vi "SpectrometerSpinCoater_v07.vi"() -> ()   [LabVIEW 2018]
uses:
  <instrlib>/Classes/CCD/Abstract_CCD/Abstract_CCD.lvclass
  <instrlib>/Classes/SpinCoater/SpinCoater.lvclass
  TypDef/DeviceQueue_TypeDef.ctl
  TypDef/DeviceQueue_Action.ctl
  TypDef/DataQueue_TypeDef.ctl
  TypDef/DataQueue_Action.ctl
  <vilib>/Utility/error.llb/DialogType.ctl
  <instrlib>/Classes/CCD/Avantes/Avantes.lvclass
  C:/Program Files/National Instruments/LabVIEW 2018/instr.lib/Classes/CCD/Abstract_CCD/Abstract_CCD.lvclass
  <vilib>/Analysis/baseanly.llb/A x Vector.vi
  <vilib>/Analysis/NI_AALBase.lvlib
panel:
  out "Time.spin":refnum<file>
  out "Meas.spin":refnum<file>
  out "Arduino":bool
  out "NKT":bool
  out "Spectromter":bool
  in  "Abort Button":bool
  in  "Stop Button":bool
  in  "Tab Control":enum32{"Measure", "Settings"}(tab)
  in  "Program Spin Coater":T1(array[cluster])
  in  "Spectra Count":u16
  in  "Measure Spectrum":bool
  out "Action":string
  out "Overall Time":dbl
  in  "Seconds after Spin Stop":dbl[unit]=0.5
  in  "Seconds to Spin Start":dbl[unit]=1.0
  in  "Calculate Frames":bool=TRUE
  in  "Frames":i32
  in  "StartMeasurement_Button":bool
  in  "Preview":bool
  out "XY Graph":T2(graph)
  in  "Frames for Spectrometer":dbl=1.0
  in  "StartSpin_Button":bool
  in  "Record RefSpec":bool
  in  "Record_Darkspec":bool
  in  "Comments":string="Just for testing"
  in  "File Name":string="Temp"
  in  "Save Path":path=path "C:/Users/Timo/Desktop/SpinCoater/Measurement"
  out "Frame Rate":dbl[unit]
  in  "Integration Time":dbl[unit]=3e-05
  in  "Dividider Get Spectra":u32=1 min=1
  in  "Automatically \nadjust count":bool=TRUE
  in  "Reset Count\nafter Spin Coating":bool=TRUE
  in  "Speed":dbl
  in  "Milliseconds":dbl
  in  "Debug":bool
  in  "Port Arduino":refnum<visa-resource-name>="COM6"
  out "Error Arduino":bool caption="Error"
  in  "Init_Arduino":bool=TRUE caption="Init"
  out "Caption_Settings_Arduino":string="Arduino"
  out "Caption_Settings_NKT":string="NKT Laser"
  out "Error_Spectromter":bool caption="Error"
  in  "Init_Spectrometer":bool=TRUE caption="Init"
  out "Caption_Settings_Spectrometer":string="Spectromter"
  # "Speed (rpm)   Time (s)        Acceleration \n                                               (rpm/s)"
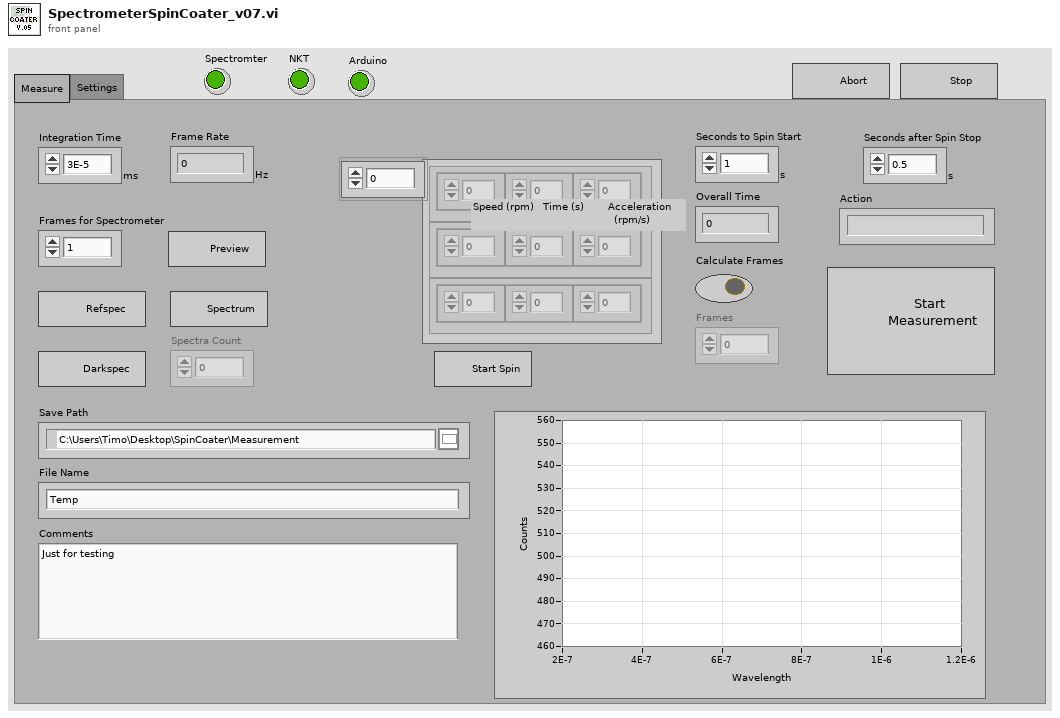
[diagram p1: front panel]
types:
  T1 = cluster{"Speed (rpm)":dbl, "Time (s)":dbl, "Acc (rpm/s)":dbl}[]
  T2 = cluster{"Wavlength":dbl[unit][], "Image":dbl[]}[]
  T3 = cluster{"Dark":cluster{"Image":dbl[][][], "Frame Size":cluster{"F":i32, "Y":i32, "X":i32}}[], "Ref":cluster{"Image":dbl[][][], "Frame Size":cluster{"F":i32, "Y":i32, "X":i32}}[], "Wavlength":dbl[unit][], "spec":dbl[][]}
  T4 = cluster{"Abstract_CCD.lvclass":refnum<class "Abstract_CCD.lvclass">, "SpinCoater.lvclass":refnum<class "SpinCoater.lvclass">}
  T5 = typedef "DataQueue_TypeDef.ctl" = cluster{"QueueAction":T6, "Data":cluster{"Image":dbl[][][], "Frame Size":cluster{"F":i32, "Y":i32, "X":i32}}[], "Data_Raw":cluster{"Image":dbl[][][], "Frame Size":cluster{"F":i32, "Y":i32, "X":i32}}[], "Data_Dark":cluster{"Image":dbl[][][], "Frame Size":cluster{"F":i32, "Y":i32, "X":i32}}[], "Data_Ref":cluster{"Image":dbl[][][], "Frame Size":cluster{"F":i32, "Y":i32, "X":i32}}[], "Device Information":string[], "Numeric Control":dbl, "Boolean":bool, "Wavelength":dbl[unit][], "Time":dbl[], "Time Stamp":timestamp, "Numeric Control 2":dbl}
  T6 = typedef "DataQueue_Action.ctl" = enum16{"TimeOut", "Close_Program", "Stop_Measurement", "Measure_InSituSpinCoating", "Measure_Spectrum", "Save_Data", "Set_Ref", "Set_Dark", "Set_Wavelength", "Spectrometer_Measure", "Spectrometer_Preview", "Transfer_Settings"}
  T7 = typedef "DeviceQueue_TypeDef.ctl" = cluster{"QueueAction":T8, "Numeric 1":dbl, "Numeric 2":dbl, "Boolean 1":bool, "Boolean 2":bool, "Spin Program":dbl[][], "Spin Prg v07":cluster{"Speed (rpm)":dbl, "Time (s)":dbl, "Acc (rpm/s)":dbl}[]}
  T8 = typedef "DeviceQueue_Action.ctl" = enum16{"TimeOut", "Close_Program", "Abort", "Spectrometer_Init", "Spectrometer_Close", "Spectrometer_DeviceInformation", "Spectrometer_Measure", "Spectrometer_Preview", "Spectrometer_Abort", "Spectrometer_StartMeasurement", "Spectrometer_GetData", "Spectrometer_StopMeasurement", "Spectrometer_SetIntegrationTime", "Spectrometer_SetFrames", "Spectrometer_SetDarkspec", "Spectrometer_SetReference", "Spectrometer_SetTriggerMode", "Laser_Init", "Laser_Close", "Arduino_Init", "Arduino_Close", "Arduino_LoadProgram", "Arduino_StartProgram", "Arduino_SetSpeed", "Arduino_SetMillis", "Arduino_StopSpin", "Measure_InSitu", "Measure_Spectrum", "Measure_Stop"}
  T9 = enum16{"open", "replace", "create", "open or create", "replace or create", "replace or create with confirmation"}
  T10 = cluster{"Image":dbl[][][], "Frame Size":cluster{"F":i32, "Y":i32, "X":i32}}[]
  T11 = cluster{"Image":dbl[][][], "Frame Size":cluster{"F":i32, "Y":i32, "X":i32}}
  T12 = cluster{"Wavlength":dbl[unit][], "A x Vector":dbl[]}
  T13 = cluster{"Wavlength":dbl[unit][], "A x Vector":dbl[]}[]
  T14 = cluster{u16[][], u16[][], dbl[], "Numeric Control":dbl, "Numeric Control 2":dbl}
  T15 = typedef "DialogType.ctl" = u16
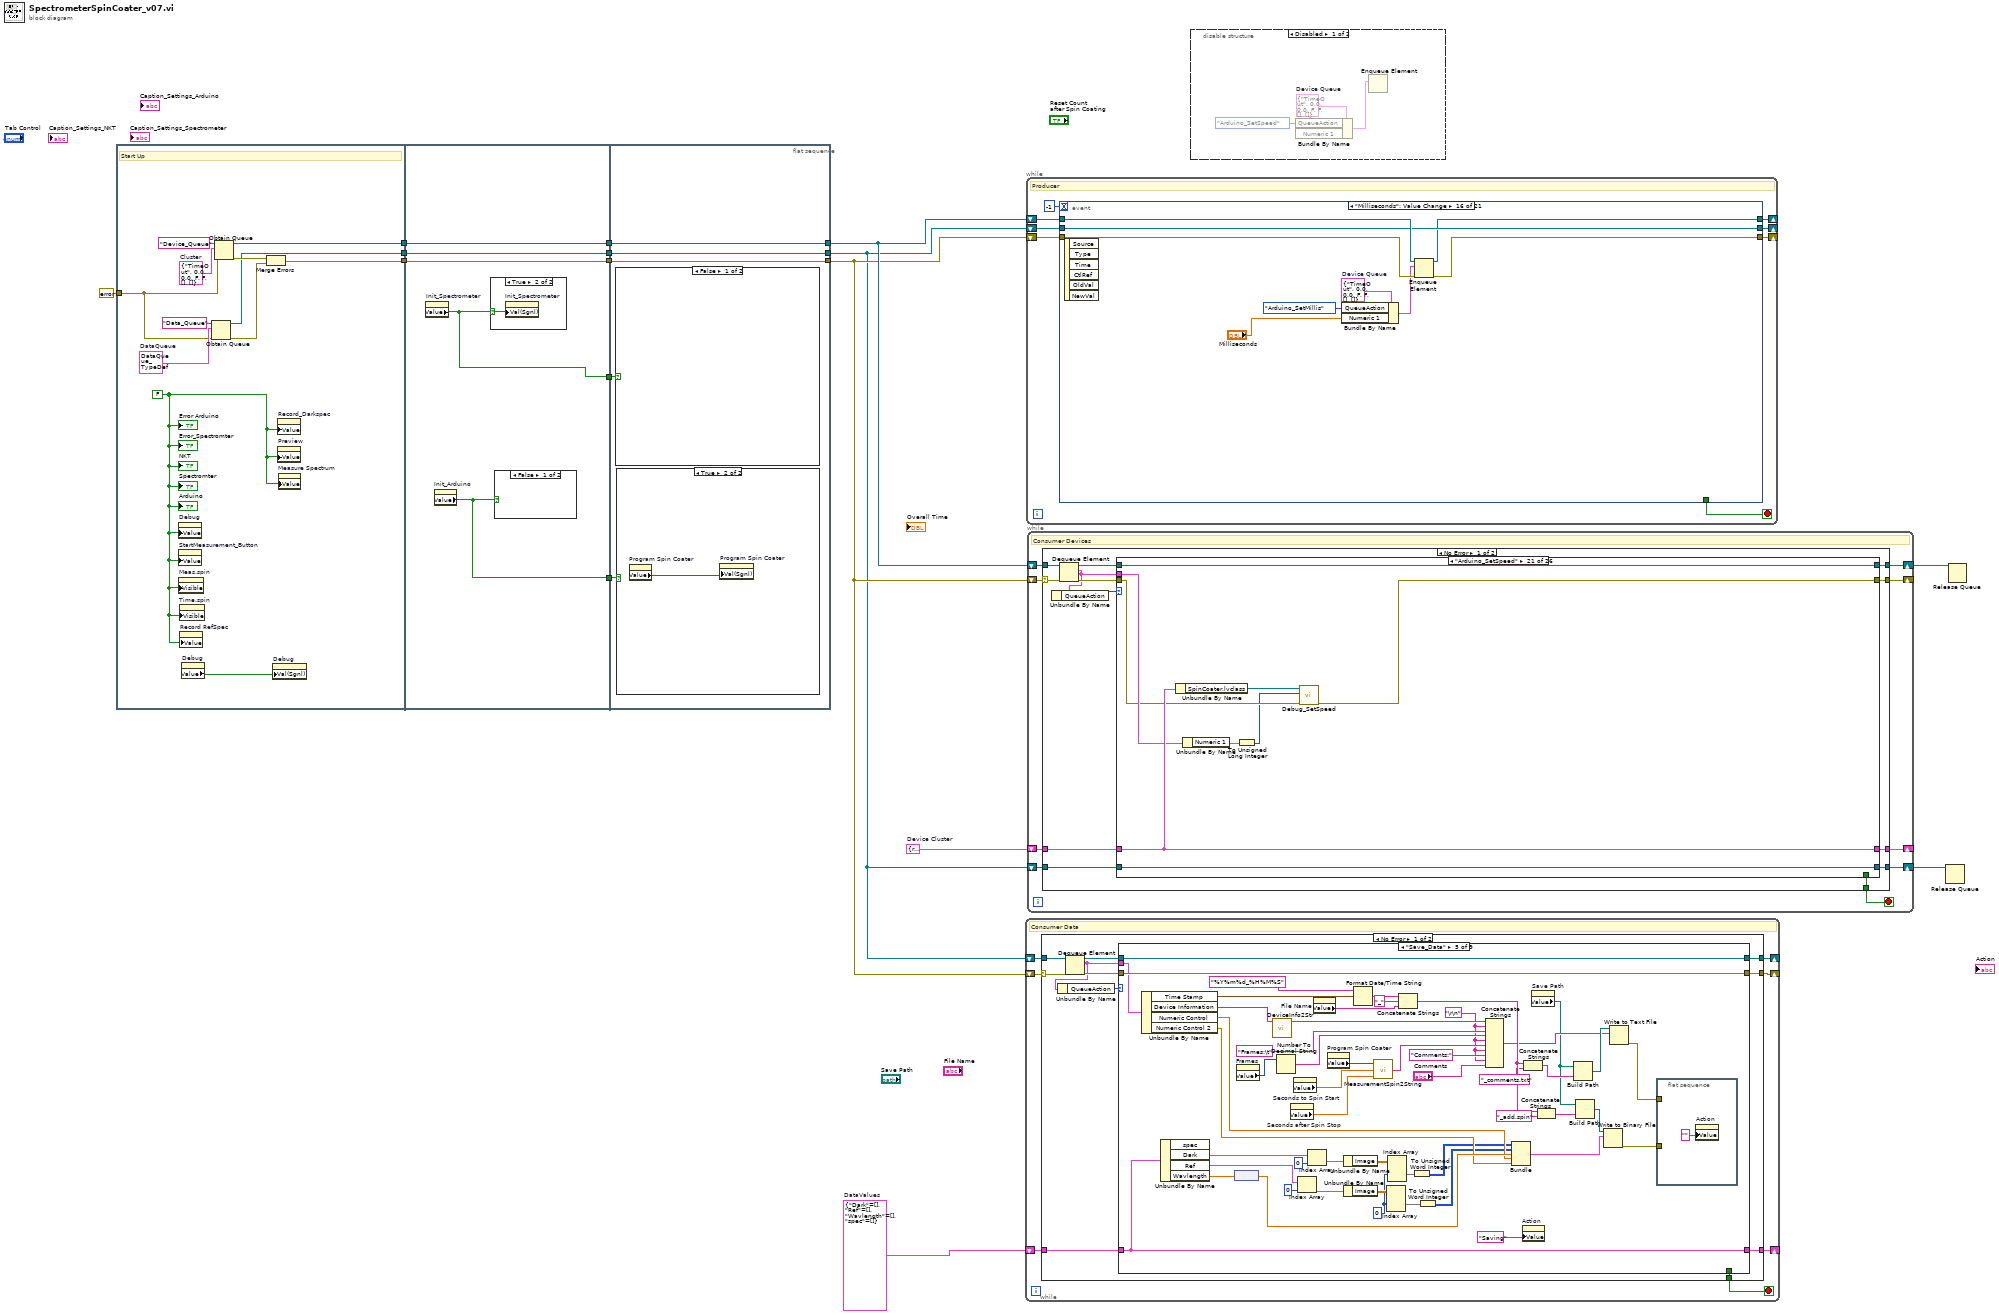
[diagram p0: block diagram]
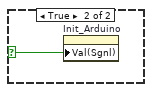
[diagram p3: hidden frame]
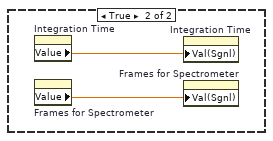
[diagram p6: hidden frame]
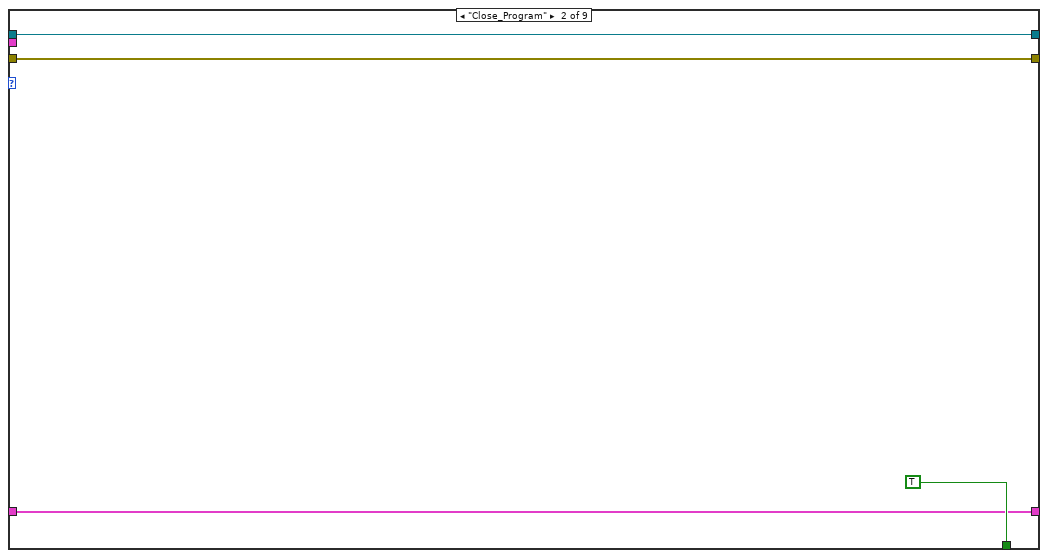
[diagram p8: hidden frame]
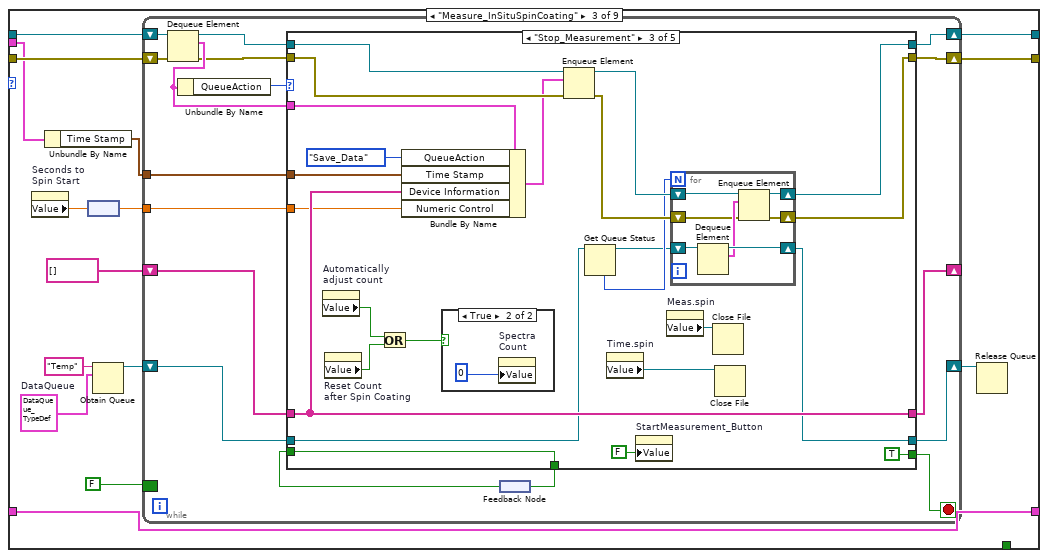
[diagram p9: hidden frame]
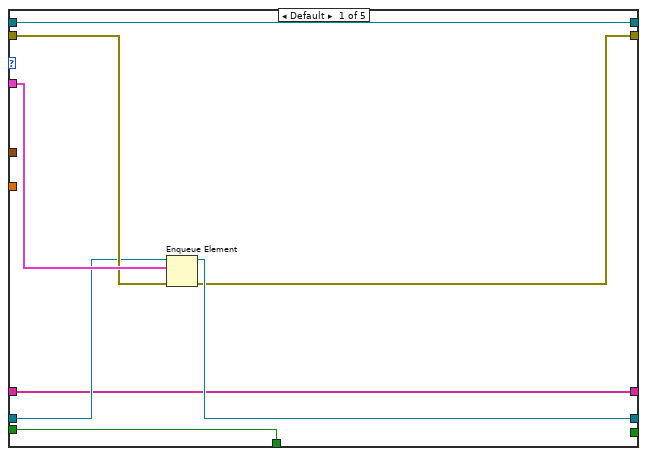
[diagram p10: hidden frame]
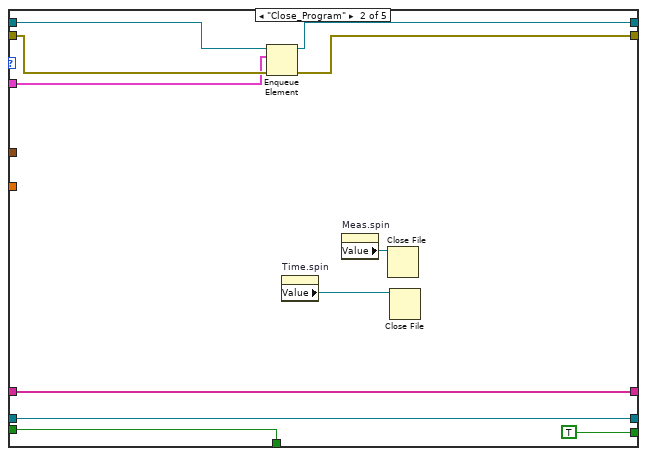
[diagram p11: hidden frame]
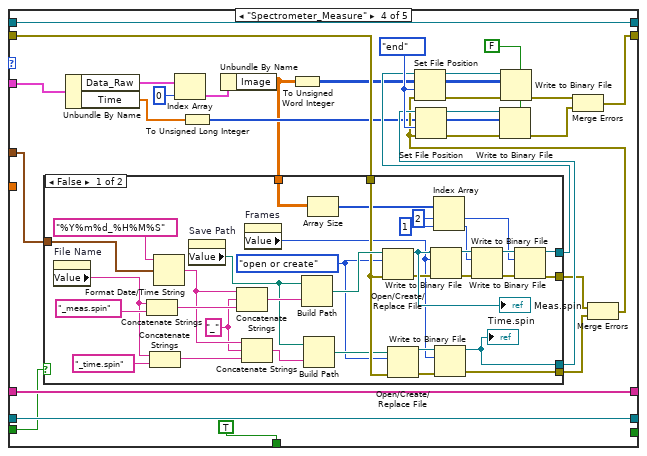
[diagram p13: hidden frame]
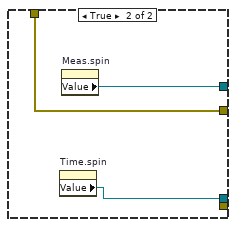
[diagram p14: hidden frame]
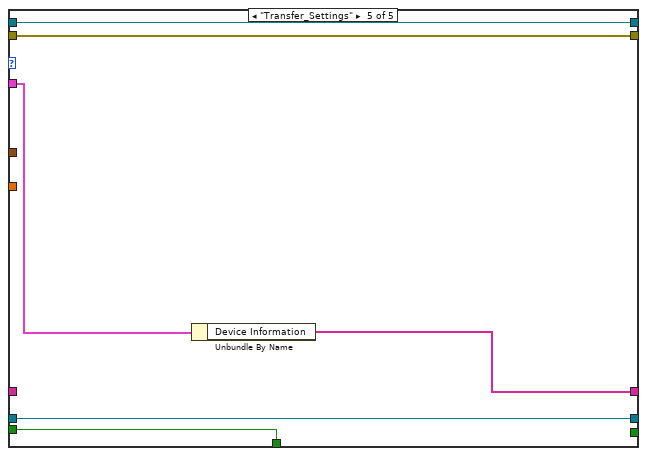
[diagram p15: hidden frame]
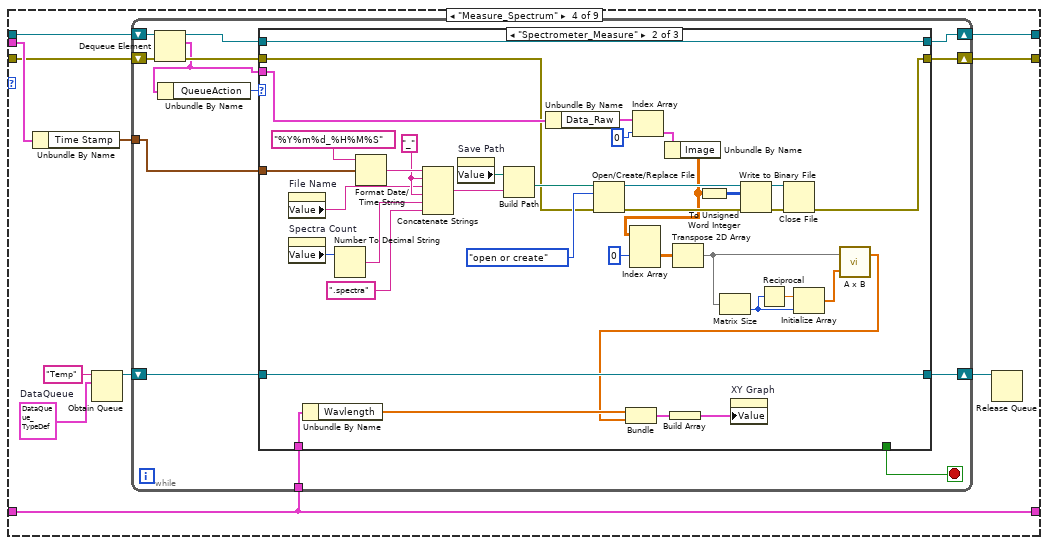
[diagram p16: hidden frame]
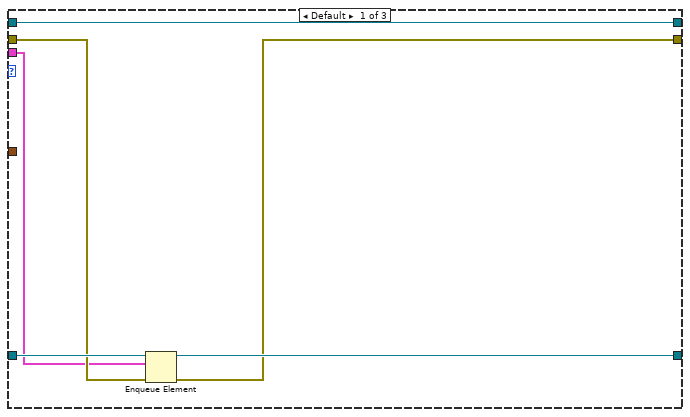
[diagram p17: hidden frame]
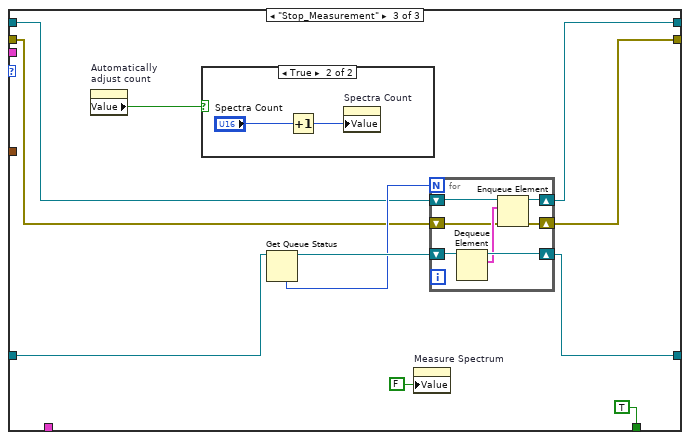
[diagram p18: hidden frame]
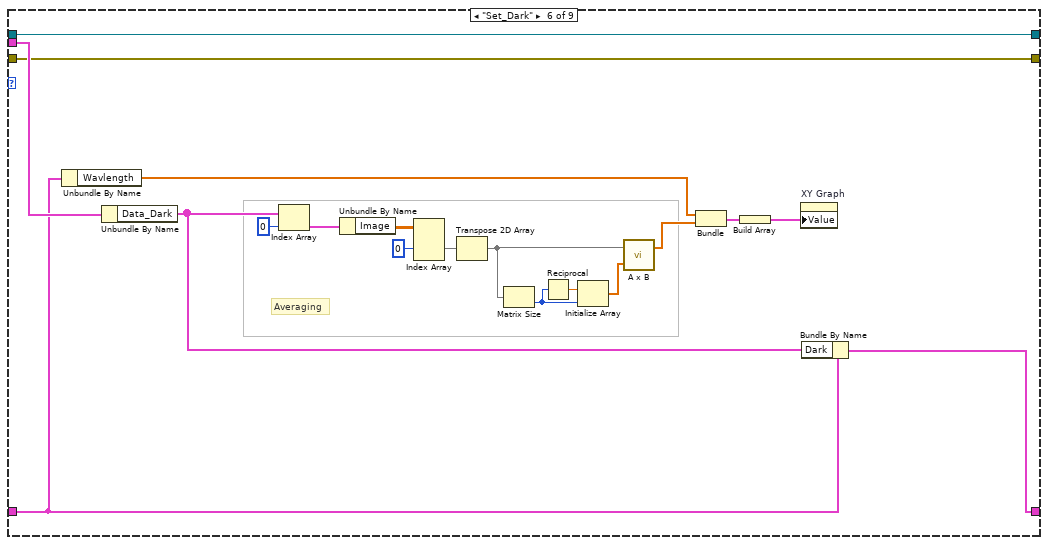
[diagram p20: hidden frame]
diagram:
  w6 = T3 {"Dark"=[], "Ref"=[], "Wavlength"=[], "spec"=[]}  # DataValues
  w11 = T4 {"Abstract_CCD.lvclass"=refnum, "SpinCoater.lvclass"=refnum}  # Device Cluster
  n1 = flat-sequence {
    tunnel: errorcluster {"status"=FALSE, "code"=0, "source"=""} ("error constant") -> [w23]
    tunnel: [w26] -> w15
    tunnel: [w20] -> w14
    tunnel: [w19] -> w13
    tunnel: w15 -> [w33]
    tunnel: w14 -> [w32]
    tunnel: w13 -> [w31]
    tunnel: [w33] -> w5
    tunnel: [w32] -> w4
    tunnel: [w31] -> w3
    tunnel: [w30] -> w2
    tunnel: [w29] -> w1
    tunnel: [w38] -> w8
    tunnel: [w39] -> w7
    tunnel: [w40] -> w12
    tunnel: w5 -> [w40]
    tunnel: w4 -> [w39]
    tunnel: w3 -> [w38]
    tunnel: w2 -> [w37]
    tunnel: w1 -> [w36]
    frame #0 {
      w24 = T5 {"QueueAction"=enum."TimeOut", "Data"=[], "Data_Raw"=[], "Data_Dark"=[], "Data_Ref"=[], "Device Information"=[], "Numeric Control"=0.0, "Boolean"=FALSE, "Wavelength"=[], "Time"=[], "Time Stamp"=timestamp(0 s since 1904-01-01), "Numeric Control 2"=0.0}  # DataQueue
      w27 = T7 {"QueueAction"=enum."TimeOut", "Numeric 1"=0.0, "Numeric 2"=0.0, "Boolean 1"=FALSE, "Boolean 2"=FALSE, "Spin Program"=[], "Spin Prg v07"=[]}  # Cluster
      w18 = FALSE ("Error Arduino")
      # "Start Up"
      n2 = property on="Debug" class="Bool (strict)"("Value"=w18) -> ()  [unwired: 2 in, 2 out]
      n3 = property on="StartMeasurement_Button" class="Bool (strict)"("Value"=w18) -> ()  [unwired: 2 in, 2 out]
      n4 = property on="Meas.spin" class="Ref (strict)"("Visible"=w18) -> ()  [unwired: 2 in, 2 out]
      n5 = property on="Time.spin" class="Ref (strict)"("Visible"=w18) -> ()  [unwired: 2 in, 2 out]
      n6 = property on="Record RefSpec" class="Bool (strict)"("Value"=w18) -> ()  [unwired: 2 in, 2 out]
      n7 = property on="Debug" class="Bool (strict)"() -> ("Value"=w17:bool)  [unwired: 2 in, 2 out]
      n8 = Obtain Queue(name (unnamed)="Data_Queue", element data type=w24, error in (no error)=w23) -> (queue out=w20:refnum<queue>, error out=w21:errorcluster)  [unwired: 2 in, 1 out]
      n9 = Obtain Queue(name (unnamed)="Device_Queue", element data type=w27, error in (no error)=w23) -> (queue out=w26:refnum<queue>, error out=w22:errorcluster)  [unwired: 2 in, 1 out]
      n10 = Merge Errors(w22, w21) -> (w19:errorcluster)
      n11 = property on="Debug" class="Bool (strict)"("Val(Sgnl)"=w17) -> ()  [unwired: 2 in, 2 out]
      n12 = property on="Record_Darkspec" class="Bool (strict)"("Value"=w18) -> ()  [unwired: 2 in, 2 out]
      n13 = property on="Preview" class="Bool (strict)"("Value"=w18) -> ()  [unwired: 2 in, 2 out]
      n14 = property on="Measure Spectrum" class="Bool (strict)"("Value"=w18) -> ()  [unwired: 2 in, 2 out]
      "Error_Spectromter" <- w18
      "Error Arduino" <- w18
      "Spectromter" <- w18
      "NKT" <- w18
      "Arduino" <- w18
    }
    frame #1 {
      n15 = property on="Init_Spectrometer" class="Bool (strict)"() -> ("Value"=w30:bool)  [unwired: 2 in, 2 out]
      n16 = property on="Init_Arduino" class="Bool (strict)"() -> ("Value"=w29:bool)  [unwired: 2 in, 2 out]
      n17 = case shown="True" w30 {
        selector: w30 -> [_ w35]
        frame False {
        }
        frame True {
          n18 = property on="Init_Spectrometer" class="Bool (strict)"("Val(Sgnl)"=w35) -> ()  [unwired: 2 in, 2 out]
        }
      }
      n19 = case shown="False" w29 {
        selector: w29 -> [_ w34]
        frame False {
        }
        frame True {
          n20 = property on="Init_Arduino" class="Bool (strict)"("Val(Sgnl)"=w34) -> ()  [unwired: 2 in, 2 out]
        }
      }
    }
    frame #2 {
      n21 = case shown="False" w37 {
        frame False {
        }
        frame True {
          n22 = property on="Integration Time" class="DigNum (strict)"() -> ("Value"=w42:dbl[unit])  [unwired: 2 in, 2 out]
          n23 = property on="Frames for Spectrometer" class="DigNum (strict)"() -> ("Value"=w43:dbl)  [unwired: 2 in, 2 out]
          n24 = property on="Integration Time" class="DigNum (strict)"("Val(Sgnl)"=w42) -> ()  [unwired: 2 in, 2 out]
          n25 = property on="Frames for Spectrometer" class="DigNum (strict)"("Val(Sgnl)"=w43) -> ()  [unwired: 2 in, 2 out]
        }
      }
      n26 = case shown="True" w36 {
        frame False {
        }
        frame True {
          n27 = property on="Program Spin Coater" class="Arr (strict)"() -> ("Value"=w41:T1)  [unwired: 2 in, 2 out]
          n28 = property on="Program Spin Coater" class="Arr (strict)"("Val(Sgnl)"=w41) -> ()  [unwired: 2 in, 2 out]
        }
      }
    }
  }
  n29 = while {
    shift-right: [w44] -> _
    shift-left: w8 -> [w50]
    shift-right: [w45] -> _
    shift-left: w7 -> [w49]
    shift-right: [w46] -> _
    shift-left: w6 -> [w48]
    stop <- w47 stop-if-true
    # "Consumer Data"
    n30 = case shown="No Error" w50 {
      selector: w50 -> [w61 w423]
      tunnel: w49 -> [w60 w424]
      tunnel: w48 -> [w58 w421]
      tunnel: [w57 _] -> w47
      tunnel: [w56 w421] -> w46
      tunnel: [w55 w424] -> w45
      tunnel: [w53 w422] -> w44
      frame No Error {
        n31 = Dequeue Element(queue=w60, error in (no error)=w61) -> (queue out=w54:refnum<queue>, element=w51:T5, error out=w52:errorcluster)  [unwired: 1 in, 1 out]
        n32 = Unbundle By Name(w51) -> ("QueueAction"=w59:T6)
        n33 = case shown="\"Save_Data\"" w59 {
          tunnel: w58 -> [w62 w67 w73 w225 w335 w375 w384 w406 w417]
          tunnel: [_ TRUE _ _ _ _ _ _ _] -> w57
          tunnel: [w62 w67 w73 w225 w335 w379 w398 w405 w417] -> w56
          tunnel: [w64 w66 w83 w231 w362 w380 w399 w402 w420] -> w55
          tunnel: w54 -> [w64 w66 w81 w233 w362 w380 w399 w402 w420]
          tunnel: [w63 w65 w82 w230 w361 w381 w400 w403 w419] -> w53
          tunnel: w52 -> [w63 w65 w80 w234 w361 w381 w400 w403 w419]
          tunnel: w51 -> [_ _ w75 w235 w348 w382 w401 w404 w418]
          frame "TimeOut", Default {
          }
          frame "Close_Program" {
          }
          frame "Measure_InSituSpinCoating" {
            w78 = T5 {"QueueAction"=enum."TimeOut", "Data"=[], "Data_Raw"=[], "Data_Dark"=[], "Data_Ref"=[], "Device Information"=[], "Numeric Control"=0.0, "Boolean"=FALSE, "Wavelength"=[], "Time"=[], "Time Stamp"=timestamp(0 s since 1904-01-01), "Numeric Control 2"=0.0}  # DataQueue
            n34 = property on="Seconds to\nSpin Start" class="DigNum (strict)"() -> ("Value"=w70:dbl[unit])  [unwired: 2 in, 2 out]
            n35 = Unbundle By Name(w75) -> ("Time Stamp"=w74:timestamp)
            n36 = node(w70) -> (w69:dbl)
            n37 = Obtain Queue(name (unnamed)="Temp", element data type=w78) -> (queue out=w77:refnum<queue>)  [unwired: 3 in, 2 out]
            n38 = while {
              shift-right: [w91] -> w83
              shift-left: w81 -> [w100]
              shift-right: [w92] -> w82
              shift-left: w80 -> [w99]
              shift-right: [w93] -> w76
              shift-left: w77 -> [w94]
              tunnel: w74 -> [w87]
              shift-right: [w88] -> _
              shift-left: string[] [] ("Device Information") -> [w89]
              border: FALSE -> [_]
              tunnel: w69 -> [w84]
              stop <- w90 stop-if-true
              n39 = Dequeue Element(queue=w100, error in (no error)=w99) -> (queue out=w95:refnum<queue>, element=w97:T5, error out=w96:errorcluster)  [unwired: 1 in, 1 out]
              n40 = Unbundle By Name(w97) -> ("QueueAction"=w98:T6)
              n41 = feedback #1() -> (w86:bool)
              n42 = case shown="\"Stop_Measurement\"" w98 {
                tunnel: w97 -> [w108 w117 w142 w179 w223]
                tunnel: w96 -> [w107 w118 w139 w170 w220]
                tunnel: w95 -> [w103 w119 w138 w178 w221]
                tunnel: w94 -> [w106 w114 w133 w167 w224]
                tunnel: [w105 w114 w130 w167 w224] -> w93
                tunnel: [w104 w115 w129 w168 w220] -> w92
                tunnel: [w103 w116 w128 w178 w221] -> w91
                tunnel: [_ TRUE TRUE _ _] -> w90
                tunnel: w89 -> [w102 w112 w140 w165 _]
                tunnel: [w102 w112 w140 w165 w222] -> w88
                tunnel: w87 -> [_ _ w141 w180 _]
                tunnel: w86 -> [w101 w111 w127 w163 w219]
                tunnel: [w101 w111 w127 TRUE w219] -> w85
                tunnel: w84 -> [_ _ w124 _ _]
                frame Default {
                  n43 = Enqueue Element(queue=w106, element=w108, error in (no error)=w107) -> (queue out=w105:refnum<queue>, error out=w104:errorcluster)  [unwired: 1 in, 1 out]
                }
                frame "Close_Program" {
                  n44 = Enqueue Element(queue=w119, element=w117, error in (no error)=w118) -> (queue out=w116:refnum<queue>, error out=w115:errorcluster)  [unwired: 1 in, 1 out]
                  n45 = property on="Time.spin" class="Ref (strict)"() -> ("Value"=w109:refnum<file>)  [unwired: 2 in, 2 out]
                  n46 = property on="Meas.spin" class="Ref (strict)"() -> ("Value"=w110:refnum<file>)  [unwired: 2 in, 2 out]
                  n47 = Close File(refnum=w110) -> ()  [unwired: 1 in, 2 out]
                  n48 = Close File(refnum=w109) -> ()  [unwired: 1 in, 2 out]
                }
                frame "Stop_Measurement" {
                  n49 = property on="Automatically \nadjust count" class="Bool (strict)"() -> ("Value"=w121:bool)  [unwired: 2 in, 2 out]
                  n50 = property on="Reset Count\nafter Spin Coating" class="Bool (strict)"() -> ("Value"=w122:bool)  [unwired: 2 in, 2 out]
                  n51 = Or(x=w121, y=w122) -> (x .or. y?=w120:bool)
                  n52 = Bundle By Name(cluster=w142, "QueueAction"=DataQueue_Action."Save_Data", "Time Stamp"=w141, "Device Information"=w140, "Numeric Control"=w124) -> (w137:T5)
                  n53 = case shown="True" w120 {
                    frame False {
                    }
                    frame True {
                      n54 = property on="Spectra \nCount" class="DigNum (strict)"("Value"=u16 0 ("Spectra Count")) -> ()  [unwired: 2 in, 2 out]
                    }
                  }
                  n55 = Enqueue Element(queue=w138, element=w137, error in (no error)=w139) -> (queue out=w135:refnum<queue>, error out=w134:errorcluster)  [unwired: 1 in, 1 out]
                  n56 = Get Queue Status(queue=w133) -> (queue out=w131:refnum<queue>, # elements in queue=w132:i32)  [unwired: 2 in, 6 out]
                  n57 = property on="Time.spin" class="Ref (strict)"() -> ("Value"=w125:refnum<file>)  [unwired: 2 in, 2 out]
                  n58 = property on="StartMeasurement_Button" class="Bool (strict)"("Value"=FALSE ("StartMeasurement_Button")) -> ()  [unwired: 2 in, 2 out]
                  n59 = property on="Meas.spin" class="Ref (strict)"() -> ("Value"=w126:refnum<file>)  [unwired: 2 in, 2 out]
                  n60 = for {
                    N: w132 -> [_]
                    shift-right: [w150] -> w130
                    shift-left: w131 -> [w151]
                    shift-right: [w147] -> w128
                    shift-left: w135 -> [w148]
                    shift-right: [w145] -> w129
                    shift-left: w134 -> [w146]
                    n61 = Dequeue Element(queue=w151) -> (queue out=w150:refnum<queue>, element=w149:T5)  [unwired: 2 in, 2 out]
                    n62 = Enqueue Element(queue=w148, element=w149, error in (no error)=w146) -> (queue out=w147:refnum<queue>, error out=w145:errorcluster)  [unwired: 1 in, 1 out]
                  }
                  n63 = Close File(refnum=w126) -> ()  [unwired: 1 in, 2 out]
                  n64 = Close File(refnum=w125) -> ()  [unwired: 1 in, 2 out]
                }
                frame "Spectrometer_Measure" {
                  w153 = FALSE ("prepend array or string size? (T)")
                  w166 = enum16{"start", "end", "current"}."end" ("from (0:start)")
                  n65 = Unbundle By Name(w179) -> ("Data_Raw"=w175:T10, "Time"=w169:dbl[])
                  n66 = Index Array(array=w175, index=0) -> (element=w174:T11)
                  n67 = To Unsigned Long Integer(number=w169) -> (unsigned 32bit integer=w155:u32[])
                  n68 = Unbundle By Name(w174) -> ("Image"=w152:dbl[][][])
                  n69 = case shown="False" w163 {
                    tunnel: w180 -> [w212 _]
                    tunnel: w170 -> [w207 w218]
                    tunnel: [w193 w218] -> w157
                    tunnel: [w181 _] -> w158
                    tunnel: [w192 w217] -> w160
                    tunnel: [w182 w216] -> w159
                    tunnel: w152 -> [w190 _]
                    frame False {
                      w202 = T9."open or create" ("operation (0:open)")
                      w201 = "_" ("string")
                      n70 = property on="File Name" class="Str"() -> ("Value"=w210:string)  [unwired: 2 in, 2 out]
                      n71 = Concatenate Strings(w210, "_meas.spin" ("string")) -> (w213:string)
                      n72 = Concatenate Strings(w210, "_time.spin" ("string")) -> (w205:string)
                      n73 = Format Date/Time String(time format string (%c)="%Y%m%d_%H%M%S", seconds (now)=w212) -> (date/time string=w206:string)  [unwired: 1 in]
                      n74 = property on="Save Path" class="Path"() -> ("Value"=w184:path)  [unwired: 2 in, 2 out]
                      n75 = Concatenate Strings(w206, w201, w213) -> (w211:string)
                      n76 = Concatenate Strings(w206, w201, w205) -> (w204:string)
                      n77 = property on="Frames" class="DigNum (strict)"() -> ("Value"=w183:i32)  [unwired: 2 in, 2 out]
                      n78 = Build Path(base path=w184, name or relative path=w211) -> (appended path=w208:path)
                      n79 = Build Path(base path=w184, name or relative path=w204) -> (appended path=w203:path)
                      n80 = Array Size(array=w190) -> (size(s)=w189:i32[])
                      n81 = Open/Create/Replace File(file path (use dialog)=w208, error in=w207, operation (0:open)=w202) -> (refnum out=w200:refnum<file>, error out=w199:errorcluster)  [unwired: 3 in, 1 out]
                      "Meas.spin" <- w200
                      n82 = Open/Create/Replace File(file path (use dialog)=w203, error in=w207, operation (0:open)=w202) -> (refnum out=w198:refnum<file>, error out=w197:errorcluster)  [unwired: 3 in, 1 out]
                      n83 = Write to Binary File(file (use dialog)=w200, data=w183, error in=w199) -> (refnum out=w196:refnum<file>, error out=w195:errorcluster)  [unwired: 3 in, 1 out]
                      n84 = Index Array(array=w189, index #1=2 ("index"), index #2=1 ("index")) -> (element #1=w185:i32, element #2=w186:i32)
                      n85 = Write to Binary File(file (use dialog)=w198, data=w183, error in=w197) -> (refnum out=w182:refnum<file>, error out=w181:errorcluster)  [unwired: 3 in, 1 out]
                      "Time.spin" <- w182
                      n86 = Write to Binary File(file (use dialog)=w196, data=w186, error in=w195) -> (refnum out=w191:refnum<file>, error out=w194:errorcluster)  [unwired: 3 in, 1 out]
                      n87 = Write to Binary File(file (use dialog)=w191, data=w185, error in=w194) -> (refnum out=w192:refnum<file>, error out=w193:errorcluster)  [unwired: 3 in, 1 out]
                    }
                    frame True {
                      n88 = property on="Time.spin" class="Ref (strict)"() -> ("Value"=w216:refnum<file>)  [unwired: 2 in, 2 out]
                      n89 = property on="Meas.spin" class="Ref (strict)"() -> ("Value"=w217:refnum<file>)  [unwired: 2 in, 2 out]
                    }
                  }
                  n90 = To Unsigned Word Integer(number=w152) -> (unsigned 16bit integer=w154:u16[][][])
                  n91 = Merge Errors(w157, w158) -> (w156:errorcluster)
                  n92 = Set File Position(refnum=w160, from (0:start)=w166, error in=w156) -> (refnum out=w172:refnum<file>, error out=w171:errorcluster)  [unwired: 1 in]
                  n93 = Set File Position(refnum=w159, from (0:start)=w166, error in=w156) -> (refnum out=w177:refnum<file>, error out=w176:errorcluster)  [unwired: 1 in]
                  n94 = Write to Binary File(file (use dialog)=w177, data=w155, error in=w176, 5:w153) -> (error out=w161:errorcluster)  [unwired: 2 in, 2 out]
                  n95 = Write to Binary File(file (use dialog)=w172, data=w154, error in=w171, 5:w153) -> (error out=w162:errorcluster)  [unwired: 2 in, 2 out]
                  n96 = Merge Errors(w162, w161) -> (w168:errorcluster)
                }
                frame "Transfer_Settings" {
                  n97 = Unbundle By Name(w223) -> ("Device Information"=w222:string[])
                }
              }
              n98 = feedback-in #1(w85) -> ()
            }
            n99 = Release Queue(queue=w76) -> ()  [unwired: 2 in, 3 out]
          }
          frame "Measure_Spectrum" {
            w228 = T5 {"QueueAction"=enum."TimeOut", "Data"=[], "Data_Raw"=[], "Data_Dark"=[], "Data_Ref"=[], "Device Information"=[], "Numeric Control"=0.0, "Boolean"=FALSE, "Wavelength"=[], "Time"=[], "Time Stamp"=timestamp(0 s since 1904-01-01), "Numeric Control 2"=0.0}  # DataQueue
            n100 = Unbundle By Name(w235) -> ("Time Stamp"=w232:timestamp)
            n101 = Obtain Queue(name (unnamed)="Temp", element data type=w228) -> (queue out=w227:refnum<queue>)  [unwired: 3 in, 2 out]
            n102 = while {
              shift-right: [w239] -> w231
              shift-left: w233 -> [w247]
              shift-right: [w240] -> w230
              shift-left: w234 -> [w248]
              tunnel: w232 -> [w237]
              shift-right: [w241] -> w226
              shift-left: w227 -> [w243]
              tunnel: w225 -> [w236]
              stop <- w238 stop-if-true
              n103 = Dequeue Element(queue=w247, error in (no error)=w248) -> (queue out=w245:refnum<queue>, element=w242:T5, error out=w244:errorcluster)  [unwired: 1 in, 1 out]
              n104 = Unbundle By Name(w242) -> ("QueueAction"=w246:T6)
              n105 = case shown="\"Spectrometer_Measure\"" w246 {
                tunnel: w245 -> [w249 w267 w298]
                tunnel: w244 -> [w252 w277 w297]
                tunnel: w243 -> [w254 w289 w300]
                tunnel: w242 -> [w250 w291 _]
                tunnel: [w253 w289 w296] -> w241
                tunnel: [w251 w268 w294] -> w240
                tunnel: [w249 w267 w295] -> w239
                tunnel: [_ _ TRUE] -> w238
                tunnel: w237 -> [_ w288 _]
                tunnel: w236 -> [_ w259 _]
                frame Default {
                  n106 = Enqueue Element(queue=w254, element=w250, error in (no error)=w252) -> (queue out=w253:refnum<queue>, error out=w251:errorcluster)  [unwired: 1 in, 1 out]
                }
                frame "Spectrometer_Measure" {
                  w285 = "_"
                  n107 = property on="File Name" class="Str"() -> ("Value"=w284:string)  [unwired: 2 in, 2 out]
                  n108 = property on="Spectra Count" class="DigNum (strict)"() -> ("Value"=w290:u16)  [unwired: 2 in, 2 out]
                  n109 = Unbundle By Name(w259) -> ("Wavlength"=w256:dbl[unit][])
                  n110 = Number To Decimal String(number=w290) -> (decimal integer string=w283:string)  [unwired: 1 in]
                  n111 = Format Date/Time String(time format string (%c)="%Y%m%d_%H%M%S", seconds (now)=w288) -> (date/time string=w286:string)  [unwired: 1 in]
                  n112 = Concatenate Strings(w286, w285, w284, w285, w283, ".spectra" ("string")) -> (w281:string)
                  n113 = property on="Save Path" class="Path"() -> ("Value"=w280:path)  [unwired: 2 in, 2 out]
                  n114 = Build Path(base path=w280, name or relative path=w281) -> (appended path=w279:path)
                  n115 = Unbundle By Name(w291) -> ("Data_Raw"=w274:T10)
                  n116 = Open/Create/Replace File(file path (use dialog)=w279, error in=w277, operation (0:open)=T9."open or create") -> (refnum out=w276:refnum<file>, error out=w275:errorcluster)  [unwired: 3 in, 1 out]
                  n117 = Index Array(array=w274, index=0) -> (element=w272:T11)
                  n118 = Unbundle By Name(w272) -> ("Image"=w260:dbl[][][])
                  n119 = Index Array(array=w260, index (dim 1)=0 ("disabled index (row)")) -> (element=w266:dbl[][])  [unwired: 2 in]
                  n120 = Transpose 2D Array(2D array=w266) -> (transposed array=w263:dbl[][])
                  n121 = To Unsigned Word Integer(number=w260) -> (unsigned 16bit integer=w271:u16[][][])
                  n122 = Matrix Size(0:w263) -> (2:w264:i32)  [unwired: 1 out]
                  n123 = Write to Binary File(file (use dialog)=w276, data=w271, error in=w275) -> (refnum out=w269:refnum<file>, error out=w270:errorcluster)  [unwired: 3 in, 1 out]
                  n124 = Reciprocal(x=w264) -> (1/x=w265:dbl)
                  n125 = Close File(refnum=w269, error in=w270) -> (error out=w268:errorcluster)  [unwired: 1 out]
                  n126 = Initialize Array(w265, w264) -> (w262:dbl[])
                  n127 = call-poly <vilib>:"A x B.vi"("Vector"=w262, "A"=w263) -> ("A x Vector"=w255:dbl[])  [unwired: 1 out]
                  n128 = Bundle("Wavlength"=w256, "A x Vector"=w255) -> (w258:T12)  [unwired: 1 in]
                  n129 = Build Array(w258) -> (w257:T13)
                  n130 = property on="XY Graph" class="XYGraph (strict)"("Value"=w257) -> ()  [unwired: 2 in, 2 out]
                }
                frame "Stop_Measurement" {
                  n131 = property on="Automatically \nadjust count" class="Bool (strict)"() -> ("Value"=w292:bool)  [unwired: 2 in, 2 out]
                  n132 = case shown="True" w292 {
                    frame False {
                    }
                    frame True {
                      n133 = Increment(x="Spectra Count") -> (x+1=w303:u16)
                      n134 = property on="Spectra Count" class="DigNum (strict)"("Value"=w303) -> ()  [unwired: 2 in, 2 out]
                    }
                  }
                  n135 = Get Queue Status(queue=w300) -> (queue out=w301:refnum<queue>, # elements in queue=w299:i32)  [unwired: 2 in, 6 out]
                  n136 = property on="Measure Spectrum" class="Bool (strict)"("Value"=FALSE ("Measure Spectrum")) -> ()  [unwired: 2 in, 2 out]
                  n137 = for {
                    N: w299 -> [_]
                    shift-right: [w310] -> w296
                    shift-left: w301 -> [w311]
                    shift-right: [w307] -> w295
                    shift-left: w298 -> [w308]
                    shift-right: [w305] -> w294
                    shift-left: w297 -> [w306]
                    n138 = Dequeue Element(queue=w311) -> (queue out=w310:refnum<queue>, element=w309:T5)  [unwired: 2 in, 2 out]
                    n139 = Enqueue Element(queue=w308, element=w309, error in (no error)=w306) -> (queue out=w307:refnum<queue>, error out=w305:errorcluster)  [unwired: 1 in, 1 out]
                  }
                }
              }
            }
            n140 = Release Queue(queue=w226) -> ()  [unwired: 2 in, 3 out]
          }
          frame "Save_Data" {
            w313 = "\r\n"
            w324 = 0 ("index (page)")
            n141 = Unbundle By Name(w348) -> ("Time Stamp"=w346:timestamp, "Device Information"=w337:string[], "Numeric Control"=w334:dbl, "Numeric Control 2"=w333:dbl)
            n142 = Unbundle By Name(w335) -> ("Dark"=w358:T10, "Ref"=w356:T10, "Wavlength"=w360:dbl[unit][])  [unwired: 1 out]
            n143 = node(w360) -> (w349:dbl[])
            n144 = property on="Frames" class="DigNum (strict)"() -> ("Value"=w320:i32)  [unwired: 2 in, 2 out]
            n145 = call "DeviceInfo2Str.vi"("Device Information"=w337) -> ("String"=w336:string)  [unwired: 10 in]
            n146 = Number To Decimal String(number=w320) -> (decimal integer string=w319:string)  [unwired: 1 in]
            n147 = property on="Seconds after Spin Stop" class="DigNum (strict)"() -> ("Value"=w316:dbl[unit])  [unwired: 2 in, 2 out]
            n148 = property on="Seconds to Spin Start" class="DigNum (strict)"() -> ("Value"=w317:dbl[unit])  [unwired: 2 in, 2 out]
            n149 = Index Array(array=w356, index=0) -> (element=w354:T11)
            n150 = Index Array(array=w358, index=0) -> (element=w355:T11)
            n151 = property on="File Name" class="Str"() -> ("Value"=w330:string)  [unwired: 2 in, 2 out]
            n152 = property on="Program Spin Coater" class="Arr (strict)"() -> ("Value"=w318:T1)  [unwired: 2 in, 2 out]
            n153 = Unbundle By Name(w355) -> ("Image"=w353:dbl[][][])
            n154 = Unbundle By Name(w354) -> ("Image"=w352:dbl[][][])
            n155 = Format Date/Time String(time format string (%c)="%Y%m%d_%H%M%S", seconds (now)=w346) -> (date/time string=w345:string)  [unwired: 1 in]
            n156 = call "MeasurementSpin2String.vi"("Seconds after Spin Stop"=w316, "Seconds to Spin Start"=w317, "Program Spin Coater"=w318) -> ("concatenated string"=w315:string)
            n157 = Index Array(array=w352, index (dim 1)=w324) -> (element=w350:dbl[][])  [unwired: 2 in]
            n158 = Index Array(array=w353, index (dim 1)=w324) -> (element=w351:dbl[][])  [unwired: 2 in]
            n159 = Concatenate Strings(w345, "_" ("string"), w330) -> (w343:string)
            n160 = To Unsigned Word Integer(number=w351) -> (unsigned 16bit integer=w323:u16[][])
            n161 = To Unsigned Word Integer(number=w350) -> (unsigned 16bit integer=w322:u16[][])
            n162 = Concatenate Strings(w336, w313, "Frames:\t" ("string"), w319, w313, w315, w313, "Comments:" ("string"), w313, "Comments") -> (w332:string)
            n163 = Bundle(w323, w322, w349, "Numeric Control"=w334, "Numeric Control 2"=w333) -> (w327:T14)  [unwired: 1 in]
            n164 = property on="Action" class="Str"("Value"="Saving" ("Action")) -> ()  [unwired: 2 in, 2 out]
            n165 = Concatenate Strings(w343, "_comments.txt" ("string")) -> (w340:string)
            n166 = property on="Save Path" class="Path"() -> ("Value"=w329:path)  [unwired: 2 in, 2 out]
            n167 = Concatenate Strings(w343, "_add.spin" ("string")) -> (w341:string)
            n168 = Build Path(base path=w329, name or relative path=w340) -> (appended path=w339:path)
            n169 = Build Path(base path=w329, name or relative path=w341) -> (appended path=w328:path)
            n170 = Write to Binary File(file (use dialog)=w328, data=w327) -> (error out=w325:errorcluster)  [unwired: 4 in, 2 out]
            n171 = Write to Text File(file (use dialog)=w339, text=w332) -> (error out=w326:errorcluster)  [unwired: 2 in, 2 out]
            n172 = flat-sequence {
              tunnel: w326 -> [_]
              tunnel: w325 -> [_]
              frame #0 {
                n173 = property on="Action" class="Str"("Value"="" ("Action")) -> ()  [unwired: 2 in, 2 out]
              }
            }
          }
          frame "Set_Dark" {
            # "Averaging"
            n174 = Unbundle By Name(w375) -> ("Wavlength"=w374:dbl[unit][])
            n175 = Unbundle By Name(w382) -> ("Data_Dark"=w372:T10)
            n176 = Index Array(array=w372, index=0) -> (element=w377:T11)
            n177 = Unbundle By Name(w377) -> ("Image"=w371:dbl[][][])
            n178 = Index Array(array=w371, index (dim 1)=0 ("disabled index (row)")) -> (element=w369:dbl[][])  [unwired: 2 in]
            n179 = Transpose 2D Array(2D array=w369) -> (transposed array=w366:dbl[][])
            n180 = Matrix Size(0:w366) -> (2:w367:i32)  [unwired: 1 out]
            n181 = Reciprocal(x=w367) -> (1/x=w368:dbl)
            n182 = Initialize Array(w368, w367) -> (w365:dbl[])
            n183 = call-poly <vilib>:"A x B.vi"("Vector"=w365, "A"=w366) -> ("A x Vector"=w364:dbl[])  [unwired: 1 out]
            n184 = Bundle("Wavlength"=w374, "A x Vector"=w364) -> (w376:T12)  [unwired: 1 in]
            n185 = Build Array(w376) -> (w373:T13)
            n186 = property on="XY Graph" class="XYGraph (strict)"("Value"=w373) -> ()  [unwired: 2 in, 2 out]
            n187 = Bundle By Name(cluster=w375, "Dark"=w372) -> (w379:T3)
          }
          frame "Set_Ref" {
            # "Averaging"
            n188 = Unbundle By Name(w384) -> ("Wavlength"=w383:dbl[unit][])
            n189 = Unbundle By Name(w401) -> ("Data_Ref"=w388:T10)
            n190 = Index Array(array=w388, index=0) -> (element=w396:T11)
            n191 = Unbundle By Name(w396) -> ("Image"=w395:dbl[][][])
            n192 = Index Array(array=w395, index (dim 1)=0 ("disabled index (row)")) -> (element=w393:dbl[][])  [unwired: 2 in]
            n193 = Transpose 2D Array(2D array=w393) -> (transposed array=w390:dbl[][])
            n194 = Matrix Size(0:w390) -> (2:w391:i32)  [unwired: 1 out]
            n195 = Reciprocal(x=w391) -> (1/x=w392:dbl)
            n196 = Initialize Array(w392, w391) -> (w389:dbl[])
            n197 = call-poly <vilib>:"A x B.vi"("Vector"=w389, "A"=w390) -> ("A x Vector"=w385:dbl[])  [unwired: 1 out]
            n198 = Bundle("Wavlength"=w383, "A x Vector"=w385) -> (w387:T12)  [unwired: 1 in]
            n199 = Build Array(w387) -> (w386:T13)
            n200 = Bundle By Name(cluster=w384, "Ref"=w388) -> (w398:T3)
            n201 = property on="XY Graph" class="XYGraph (strict)"("Value"=w386) -> ()  [unwired: 2 in, 2 out]
          }
          frame "Set_Wavelength" {
            n202 = Unbundle By Name(w404) -> ("Wavelength"=w407:dbl[unit][])
            n203 = Bundle By Name(cluster=w406, "Wavlength"=w407) -> (w405:T3)
          }
          frame "Spectrometer_Preview" {
            w412 = 0 ("index (page)")
            n204 = Unbundle By Name(w418) -> ("Data_Raw"=w416:T10)
            n205 = Unbundle By Name(w417) -> ("Wavlength"=w411:dbl[unit][])
            n206 = Index Array(array=w416, index=0) -> (element=w414:T11)
            n207 = Unbundle By Name(w414) -> ("Image"=w413:dbl[][][])
            n208 = Index Array(array=w413, index (dim 0)=w412, index (dim 1)=w412) -> (element=w410:dbl[])  [unwired: 1 in]
            n209 = Bundle("Wavlength"=w411, "Image"=w410) -> (w409:cluster{"Wavlength":dbl[unit][], "Image":dbl[]})  [unwired: 1 in]
            n210 = Build Array(w409) -> (→"XY Graph":T2)
          }
        }
      }
      frame Error {
        w426 = T15 4 items=["no dialog", "OK message", "continue or stop message", "OK message + warnings", "continue/stop + warnings"] ("type of dialog (OK msg:1)")
        n211 = call <vilib>:"General Error Handler.vi"("type of dialog (OK msg:1)"=w426, "error in (no error)"=w423) -> ("error out"=w425:errorcluster)  [unwired: 9 in, 4 out]
        n212 = call <vilib>:"Clear Errors.vi"("error in (no error)"=w425) -> ("error out"=w422:errorcluster)  [unwired: 5 in, 1 out]
      }
    }
  }
  n213 = while {
    shift-right: [w429] -> _
    shift-left: w12 -> [w427]
    shift-right: [w432] -> _
    shift-left: w7 -> [w433]
    shift-right: [w430] -> _
    shift-left: w8 -> [w431]
    stop <- w428 stop-if-true
    # "Producer"
    n214 = event shown="[15] \"Milliseconds\": Value Change" {
      selector: _ -> [_ _ _ _ _ _ _ _ _ _ _ _ _ _ _ _ _ _ _ _ _]
      dyn-events: _ -> [_ _ _ _ _ _ _ _ _ _ _ _ _ _ _ _ _ _ _ _ _]
      timeout: -1 -> [_ _ _ _ _ _ _ _ _ _ _ _ _ _ _ _ _ _ _ _ _]
      tunnel: w433 -> [w436 w451 w455 w467 w480 w495 w507 w518 w521 w528 w547 w554 w563 w571 w586 w596 w605 w613 w618 w625 w637]
      tunnel: [w436 w448 w455 w467 w480 w495 w507 w518 w521 w528 w547 w554 w563 w570 w586 w596 w605 w613 w618 w623 w637] -> w432
      tunnel: w431 -> [w435 w450 w457 w465 w477 w494 w505 w513 w520 w525 w545 w553 w561 w577 w583 w595 w604 w612 w617 w630 w638]
      tunnel: [w435 w444 w454 w461 w476 w492 w503 w512 w520 w523 w544 w551 w560 w569 w584 w592 w601 w612 w617 w630 w638] -> w430
      tunnel: w427 -> [w437 w452 w458 w466 w479 w496 w506 w515 w522 w526 w548 w555 w564 w579 w587 w597 w606 w614 w619 w631 w636]
      tunnel: [w437 w449 w456 w462 w478 w493 w504 w514 w522 w527 w546 w552 w562 w578 w585 w593 w602 w614 w616 w629 w636] -> w429
      tunnel: [_ TRUE _ _ _ _ _ _ _ _ _ _ _ _ _ _ _ _ _ _ _] -> w428
      event Timeout {
        n215 = event-data() -> ()  [unwired: 1 in, 3 out]
      }
      event "Stop Button": Value Change {
        w440 = T5 {"QueueAction"=enum."TimeOut", "Data"=[], "Data_Raw"=[], "Data_Dark"=[], "Data_Ref"=[], "Device Information"=[], "Numeric Control"=0.0, "Boolean"=FALSE, "Wavelength"=[], "Time"=[], "Time Stamp"=timestamp(0 s since 1904-01-01), "Numeric Control 2"=0.0}  # DataQueue
        w443 = T7 {"QueueAction"=enum."TimeOut", "Numeric 1"=0.0, "Numeric 2"=0.0, "Boolean 1"=FALSE, "Boolean 2"=FALSE, "Spin Program"=[], "Spin Prg v07"=[]}  # Device Queue
        n216 = event-data() -> ()  [unwired: 1 in, 6 out]
        n217 = Bundle By Name(cluster=w443, "QueueAction"=DeviceQueue_Action."Close_Program") -> (w441:T7)
        n218 = Enqueue Element(queue=w452, element=w441, error in (no error)=w450) -> (queue out=w449:refnum<queue>, error out=w445:errorcluster)  [unwired: 1 in, 1 out]
        n219 = Bundle By Name(cluster=w440, "QueueAction"=DataQueue_Action."Close_Program") -> (w438:T5)
        n220 = Enqueue Element(queue=w451, element=w438, error in (no error)=w450) -> (queue out=w448:refnum<queue>, error out=w446:errorcluster)  [unwired: 1 in, 1 out]
        n221 = Merge Errors(w446, w445) -> (w444:errorcluster)
      }
      event "Abort Button": Value Change {
        w460 = T7 {"QueueAction"=enum."TimeOut", "Numeric 1"=0.0, "Numeric 2"=0.0, "Boolean 1"=FALSE, "Boolean 2"=FALSE, "Spin Program"=[], "Spin Prg v07"=[]}  # Device Queue
        # "At the moment just spin coater in non in-situ measurements can be stopped"
        n222 = event-data() -> ()  [unwired: 1 in, 6 out]
        n223 = Bundle By Name(cluster=w460, "QueueAction"=DeviceQueue_Action."Abort") -> (w459:T7)
        n224 = Enqueue Element(queue=w458, element=w459, error in (no error)=w457) -> (queue out=w456:refnum<queue>, error out=w454:errorcluster)  [unwired: 1 in, 1 out]
      }
      event "Init_Spectrometer": Value Change {
        n225 = event-data() -> ()  [unwired: 1 in, 6 out]
        n226 = case shown="True" "Init_Spectrometer" {
          tunnel: [w468 w471] -> w463
          frame True {
            n227 = Bundle By Name(cluster=T7 {"QueueAction"=enum."TimeOut", "Numeric 1"=0.0, "Numeric 2"=0.0, "Boolean 1"=FALSE, "Boolean 2"=FALSE, "Spin Program"=[], "Spin Prg v07"=[]} ("element"), "QueueAction"=DeviceQueue_Action."Spectrometer_Init") -> (w468:T7)
          }
          frame False {
            n228 = Bundle By Name(cluster=T7 {"QueueAction"=enum."TimeOut", "Numeric 1"=0.0, "Numeric 2"=0.0, "Boolean 1"=FALSE, "Boolean 2"=FALSE, "Spin Program"=[], "Spin Prg v07"=[]} ("element"), "QueueAction"=DeviceQueue_Action."Spectrometer_Close") -> (w471:T7)
          }
        }
        n229 = Enqueue Element(queue=w466, element=w463, error in (no error)=w465) -> (queue out=w462:refnum<queue>, error out=w461:errorcluster)  [unwired: 1 in, 1 out]
      }
      event "Init_Arduino": Value Change {
        n230 = event-data() -> ("NewVal"=w475:bool)  [unwired: 1 in, 5 out]
        n231 = case shown="True" w475 {
          tunnel: [w481 w484] -> w474
          frame False {
            w483 = T7 {"QueueAction"=enum."TimeOut", "Numeric 1"=0.0, "Numeric 2"=0.0, "Boolean 1"=FALSE, "Boolean 2"=FALSE, "Spin Program"=[], "Spin Prg v07"=[]}  # Device Queue
            n232 = Bundle By Name(cluster=w483, "QueueAction"=DeviceQueue_Action."Arduino_Close") -> (w481:T7)
          }
          frame True {
            w486 = T7 {"QueueAction"=enum."TimeOut", "Numeric 1"=0.0, "Numeric 2"=0.0, "Boolean 1"=FALSE, "Boolean 2"=FALSE, "Spin Program"=[], "Spin Prg v07"=[]}  # Device Queue
            n233 = Bundle By Name(cluster=w486, "QueueAction"=DeviceQueue_Action."Arduino_Init") -> (w484:T7)
          }
        }
        n234 = Enqueue Element(queue=w479, element=w474, error in (no error)=w477) -> (queue out=w478:refnum<queue>, error out=w476:errorcluster)  [unwired: 1 in, 1 out]
      }
      event "Program Spin Coater": Value Change {
        w498 = T7 {"QueueAction"=enum."TimeOut", "Numeric 1"=0.0, "Numeric 2"=0.0, "Boolean 1"=FALSE, "Boolean 2"=FALSE, "Spin Program"=[], "Spin Prg v07"=[]}  # Device Queue
        n235 = event-data() -> ("NewVal"=w487:T1)  [unwired: 1 in, 5 out]
        n236 = property on="Seconds to Spin Start" class="DigNum (strict)"() -> ("Value"=w489:dbl[unit])  [unwired: 2 in, 2 out]
        n237 = node(w489) -> (w488:dbl)
        n238 = Bundle By Name(cluster=w498, "QueueAction"=DeviceQueue_Action."Arduino_LoadProgram", "Spin Prg v07"=w487, "Numeric 1"=w488) -> (w497:T7)
        n239 = Enqueue Element(queue=w496, element=w497, error in (no error)=w494) -> (queue out=w493:refnum<queue>, error out=w492:errorcluster)  [unwired: 1 in, 1 out]
        n240 = property on="Integration Time" class="DigNum (strict)"() -> ("Value"=w490:dbl[unit])  [unwired: 2 in, 2 out]
        n241 = property on="Integration Time" class="DigNum (strict)"("Val(Sgnl)"=w490) -> ()  [unwired: 2 in, 2 out]
      }
      event "Integration Time": Value Change {
        w509 = T7 {"QueueAction"=enum."TimeOut", "Numeric 1"=0.0, "Numeric 2"=0.0, "Boolean 1"=FALSE, "Boolean 2"=FALSE, "Spin Program"=[], "Spin Prg v07"=[]}  # Device Queue
        n242 = event-data() -> ("NewVal"=w501:dbl[unit])  [unwired: 1 in, 5 out]
        n243 = node(w501) -> (w500:dbl)
        n244 = property on="Calculate Frames" class="Bool (strict)"() -> ("Value"=w499:bool)  [unwired: 2 in, 2 out]
        n245 = Bundle By Name(cluster=w509, "QueueAction"=DeviceQueue_Action."Spectrometer_SetIntegrationTime", "Numeric 1"=w500, "Boolean 1"=w499) -> (w508:T7)
        n246 = Enqueue Element(queue=w506, element=w508, error in (no error)=w505) -> (queue out=w504:refnum<queue>, error out=w503:errorcluster)  [unwired: 1 in, 1 out]
      }
      event "Frames": Value Change {
        w517 = T7 {"QueueAction"=enum."TimeOut", "Numeric 1"=0.0, "Numeric 2"=0.0, "Boolean 1"=FALSE, "Boolean 2"=FALSE, "Spin Program"=[], "Spin Prg v07"=[]}  # Device Queue
        n247 = event-data() -> ()  [unwired: 1 in, 6 out]
        n248 = Bundle By Name(cluster=w517, "QueueAction"=DeviceQueue_Action."Spectrometer_SetFrames", "Numeric 1"="Frames") -> (w516:T7)
        n249 = Enqueue Element(queue=w515, element=w516, error in (no error)=w513) -> (queue out=w514:refnum<queue>, error out=w512:errorcluster)  [unwired: 1 in, 1 out]
      }
      event "Seconds to Spin Start", "Seconds after Spin Stop": Value Change {
        n250 = event-data() -> ()  [unwired: 1 in, 6 out]
        n251 = property on="Program Spin Coater" class="Arr (strict)"() -> ("Value"=w519:T1)  [unwired: 2 in, 2 out]
        n252 = property on="Program Spin Coater" class="Arr (strict)"("Val(Sgnl)"=w519) -> ()  [unwired: 2 in, 2 out]
      }
      event "Calculate Frames": Value Change {
        n253 = event-data() -> ("NewVal"=w529:bool)  [unwired: 1 in, 5 out]
        n254 = case shown="False" w529 {
          tunnel: [0 2] -> w524
          tunnel: w526 -> [w531 w540]
          tunnel: [w531 w538] -> w527
          tunnel: w525 -> [w530 w537]
          tunnel: [w530 w533] -> w523
          frame False {
          }
          frame True {
            w539 = T7 {"QueueAction"=enum."TimeOut", "Numeric 1"=0.0, "Numeric 2"=0.0, "Boolean 1"=FALSE, "Boolean 2"=FALSE, "Spin Program"=[], "Spin Prg v07"=[]}  # Device Queue
            n255 = property on="Integration Time" class="DigNum (strict)"() -> ("Value"=w535:dbl[unit])  [unwired: 2 in, 2 out]
            n256 = node(w535) -> (w534:dbl)
            n257 = Bundle By Name(cluster=w539, "QueueAction"=DeviceQueue_Action."Spectrometer_SetIntegrationTime", "Numeric 1"=w534) -> (w541:T7)
            n258 = Enqueue Element(queue=w540, element=w541, error in (no error)=w537) -> (queue out=w538:refnum<queue>, error out=w533:errorcluster)  [unwired: 1 in, 1 out]
          }
        }
        n259 = property on="Frames" class="DigNum (strict)"("DisabledEnum"=w524) -> ()  [unwired: 2 in, 2 out]
      }
      event "Record RefSpec": Value Change {
        w550 = T7 {"QueueAction"=enum."TimeOut", "Numeric 1"=0.0, "Numeric 2"=0.0, "Boolean 1"=FALSE, "Boolean 2"=FALSE, "Spin Program"=[], "Spin Prg v07"=[]}  # Device Queue
        n260 = event-data() -> ()  [unwired: 1 in, 6 out]
        n261 = Bundle By Name(cluster=w550, "QueueAction"=DeviceQueue_Action."Spectrometer_SetReference") -> (w549:T7)
        n262 = Enqueue Element(queue=w548, element=w549, error in (no error)=w545) -> (queue out=w546:refnum<queue>, error out=w544:errorcluster)  [unwired: 1 in, 1 out]
      }
      event "Preview": Value Change {
        w558 = T7 {"QueueAction"=enum."TimeOut", "Numeric 1"=0.0, "Numeric 2"=0.0, "Boolean 1"=FALSE, "Boolean 2"=FALSE, "Spin Program"=[], "Spin Prg v07"=[]}  # Device Queue
        n263 = event-data() -> ()  [unwired: 1 in, 6 out]
        n264 = Bundle By Name(cluster=w558, "QueueAction"=DeviceQueue_Action."Spectrometer_Preview") -> (w557:T7)
        n265 = Enqueue Element(queue=w555, element=w557, error in (no error)=w553) -> (queue out=w552:refnum<queue>, error out=w551:errorcluster)  [unwired: 1 in, 1 out]
      }
      event "Record_Darkspec": Value Change {
        w566 = T7 {"QueueAction"=enum."TimeOut", "Numeric 1"=0.0, "Numeric 2"=0.0, "Boolean 1"=FALSE, "Boolean 2"=FALSE, "Spin Program"=[], "Spin Prg v07"=[]}  # Device Queue
        n266 = event-data() -> ()  [unwired: 1 in, 6 out]
        n267 = Bundle By Name(cluster=w566, "QueueAction"=DeviceQueue_Action."Spectrometer_SetDarkspec") -> (w565:T7)
        n268 = Enqueue Element(queue=w564, element=w565, error in (no error)=w561) -> (queue out=w562:refnum<queue>, error out=w560:errorcluster)  [unwired: 1 in, 1 out]
      }
      event "StartMeasurement_Button": Value Change {
        w573 = T5 {"QueueAction"=enum."TimeOut", "Data"=[], "Data_Raw"=[], "Data_Dark"=[], "Data_Ref"=[], "Device Information"=[], "Numeric Control"=0.0, "Boolean"=FALSE, "Wavelength"=[], "Time"=[], "Time Stamp"=timestamp(0 s since 1904-01-01), "Numeric Control 2"=0.0}  # DataQueue
        w581 = T7 {"QueueAction"=enum."TimeOut", "Numeric 1"=0.0, "Numeric 2"=0.0, "Boolean 1"=FALSE, "Boolean 2"=FALSE, "Spin Program"=[], "Spin Prg v07"=[]}  # Device Queue
        n269 = event-data() -> ()  [unwired: 1 in, 6 out]
        n270 = property on="Preview" class="Bool (strict)"("Value"=FALSE ("Preview")) -> ()  [unwired: 2 in, 2 out]
        n271 = Bundle By Name(cluster=w581, "QueueAction"=DeviceQueue_Action."Measure_InSitu") -> (w580:T7)
        n272 = Enqueue Element(queue=w579, element=w580, error in (no error)=w577) -> (queue out=w578:refnum<queue>, error out=w568:errorcluster)  [unwired: 1 in, 1 out]
        n273 = Get Date/Time In Seconds() -> (seconds since 1Jan1904=w567:timestamp)
        n274 = Bundle By Name(cluster=w573, "QueueAction"=DataQueue_Action."Measure_InSituSpinCoating", "Time Stamp"=w567) -> (w574:T5)
        n275 = Enqueue Element(queue=w571, element=w574, error in (no error)=w568) -> (queue out=w570:refnum<queue>, error out=w569:errorcluster)  [unwired: 1 in, 1 out]
      }
      event "StartSpin_Button": Value Change {
        w589 = T7 {"QueueAction"=enum."TimeOut", "Numeric 1"=0.0, "Numeric 2"=0.0, "Boolean 1"=FALSE, "Boolean 2"=FALSE, "Spin Program"=[], "Spin Prg v07"=[]}  # Device Queue
        n276 = event-data() -> ()  [unwired: 1 in, 6 out]
        n277 = Bundle By Name(cluster=w589, "QueueAction"=DeviceQueue_Action."Arduino_StartProgram") -> (w588:T7)
        n278 = Enqueue Element(queue=w587, element=w588, error in (no error)=w583) -> (queue out=w585:refnum<queue>, error out=w584:errorcluster)  [unwired: 1 in, 1 out]
      }
      event "Milliseconds": Value Change {
        w598 = T7 {"QueueAction"=enum."TimeOut", "Numeric 1"=0.0, "Numeric 2"=0.0, "Boolean 1"=FALSE, "Boolean 2"=FALSE, "Spin Program"=[], "Spin Prg v07"=[]}  # Device Queue
        n279 = event-data() -> ()  [unwired: 1 in, 6 out]
        n280 = Bundle By Name(cluster=w598, "QueueAction"=DeviceQueue_Action."Arduino_SetMillis", "Numeric 1"="Milliseconds") -> (w594:T7)
        n281 = Enqueue Element(queue=w597, element=w594, error in (no error)=w595) -> (queue out=w593:refnum<queue>, error out=w592:errorcluster)  [unwired: 1 in, 1 out]
      }
      event "Speed": Value Change {
        w607 = T7 {"QueueAction"=enum."TimeOut", "Numeric 1"=0.0, "Numeric 2"=0.0, "Boolean 1"=FALSE, "Boolean 2"=FALSE, "Spin Program"=[], "Spin Prg v07"=[]}  # Device Queue
        n282 = event-data() -> ()  [unwired: 1 in, 6 out]
        n283 = Bundle By Name(cluster=w607, "QueueAction"=DeviceQueue_Action."Arduino_SetSpeed", "Numeric 1"="Speed") -> (w603:T7)
        n284 = Enqueue Element(queue=w606, element=w603, error in (no error)=w604) -> (queue out=w602:refnum<queue>, error out=w601:errorcluster)  [unwired: 1 in, 1 out]
      }
      event "Debug": Value Change {
        n285 = event-data() -> ()  [unwired: 1 in, 6 out]
        n286 = Select(t=u8 0, s="Debug", f=u8 2) -> (s? t:f=w608:u8)
        n287 = property on="Milliseconds" class="DigNum (strict)"("DisabledEnum"=w608) -> ()  [unwired: 2 in, 2 out]
        n288 = property on="Speed" class="DigNum (strict)"("DisabledEnum"=w608) -> ()  [unwired: 2 in, 2 out]
      }
      event "Frames for Spectrometer": Value Change {
        w621 = T7 {"QueueAction"=enum."TimeOut", "Numeric 1"=0.0, "Numeric 2"=0.0, "Boolean 1"=FALSE, "Boolean 2"=FALSE, "Spin Program"=[], "Spin Prg v07"=[]}  # Device Queue
        n289 = event-data() -> ("NewVal"=w615:dbl)  [unwired: 1 in, 5 out]
        n290 = Bundle By Name(cluster=w621, "QueueAction"=DeviceQueue_Action."Spectrometer_SetFrames", "Numeric 1"=w615) -> (w622:T7)
        n291 = Enqueue Element(queue=w619, element=w622) -> (queue out=w616:refnum<queue>)  [unwired: 2 in, 2 out]
      }
      event "Measure Spectrum": Value Change {
        w627 = T5 {"QueueAction"=enum."TimeOut", "Data"=[], "Data_Raw"=[], "Data_Dark"=[], "Data_Ref"=[], "Device Information"=[], "Numeric Control"=0.0, "Boolean"=FALSE, "Wavelength"=[], "Time"=[], "Time Stamp"=timestamp(0 s since 1904-01-01), "Numeric Control 2"=0.0}  # DataQueue
        w633 = T7 {"QueueAction"=enum."TimeOut", "Numeric 1"=0.0, "Numeric 2"=0.0, "Boolean 1"=FALSE, "Boolean 2"=FALSE, "Spin Program"=[], "Spin Prg v07"=[]}  # Device Queue
        n292 = event-data() -> ()  [unwired: 1 in, 6 out]
        n293 = Bundle By Name(cluster=w633, "QueueAction"=DeviceQueue_Action."Measure_Spectrum") -> (w634:T7)
        n294 = Enqueue Element(queue=w631, element=w634) -> (queue out=w629:refnum<queue>)  [unwired: 2 in, 2 out]
        n295 = Get Date/Time In Seconds() -> (seconds since 1Jan1904=w628:timestamp)
        n296 = Bundle By Name(cluster=w627, "QueueAction"=DataQueue_Action."Measure_Spectrum", "Time Stamp"=w628) -> (w624:T5)
        n297 = Enqueue Element(queue=w625, element=w624) -> (queue out=w623:refnum<queue>)  [unwired: 2 in, 2 out]
      }
      event "Automatically \nadjust count": Value Change {
        n298 = event-data() -> ("NewVal"=w641:bool)  [unwired: 1 in, 5 out]
        n299 = Select(t=u8 2, s=w641, f=u8 0) -> (s? t:f=w635:u8)
        n300 = property on="Spectra Count" class="DigNum (strict)"("DisabledEnum"=w635) -> ()  [unwired: 2 in, 2 out]
      }
    }
  }
  n301 = while {
    shift-right: [w646] -> _
    shift-left: w8 -> [w650]
    shift-right: [w647] -> w10
    shift-left: w12 -> [w649]
    shift-right: [w644] -> w9
    shift-left: w7 -> [w645]
    shift-right: [w642] -> _
    shift-left: w11 -> [w643]
    stop <- w648 stop-if-true
    # "Consumer Devices"
    n302 = case shown="No Error" w650 {
      selector: w650 -> [w662 w1084]
      tunnel: w649 -> [w663 w1085]
      tunnel: [w659 _] -> w648
      tunnel: [w658 w1085] -> w647
      tunnel: [w656 w1081] -> w646
      tunnel: w645 -> [w654 w1079]
      tunnel: [w655 w1079] -> w644
      tunnel: w643 -> [w653 w1080]
      tunnel: [w652 w1080] -> w642
      frame No Error {
        n303 = Dequeue Element(queue=w663, error in (no error)=w662) -> (queue out=w661:refnum<queue>, element=w651:T7, error out=w657:errorcluster)  [unwired: 1 in, 1 out]
        n304 = Unbundle By Name(w651) -> ("QueueAction"=w660:T8)
        n305 = case shown="\"Arduino_SetSpeed\"" w660 {
          tunnel: w661 -> [w667 w687 w705 w714 w764 w778 w788 w807 w814 w833 w834 w862 w879 w894 w904 w916 w928 w949 w971 w976 w983 w995 w1001 w1011 w1057 w1076]
          tunnel: [_ w689 _ _ _ _ _ _ _ _ _ _ _ _ _ _ _ _ _ _ _ _ _ _ _ _] -> w659
          tunnel: [w667 w672 w691 w713 w764 w778 w789 w807 w814 w833 w834 w862 w879 w894 w904 w916 w927 w949 w971 w976 w983 w995 w1001 w1011 w1019 w1067] -> w658
          tunnel: w657 -> [w666 w671 w704 w725 w765 w777 w784 w810 w818 w830 w844 w860 w869 w885 w901 w912 w923 w952 w965 w973 w981 w990 w998 w1004 w1013 w1075]
          tunnel: [w666 w670 w692 w712 w759 w776 w782 w808 w815 w820 w838 w859 w866 w881 w899 w906 w926 w951 w962 w972 w979 w989 w997 w1003 w1020 w1066] -> w656
          tunnel: [w664 w669 w709 w710 w761 w773 w793 w806 w813 w824 w846 w863 w873 w888 w895 w908 w930 w950 w970 w978 w987 w993 w1002 w1006 w1028 w1074] -> w655
          tunnel: w654 -> [w664 w669 w709 w711 w761 w774 w794 w806 w813 w825 w846 w863 w876 w891 w895 w910 w930 w950 w970 w978 w987 w993 w1002 w1007 w1028 w1074]
          tunnel: w653 -> [w665 w668 w708 w722 w763 w775 w787 w805 w817 w826 w837 w856 w872 w887 w898 w905 w925 w945 w964 w977 w986 w992 w1000 w1005 w1060 w1073]
          tunnel: [w665 w668 w708 w716 w762 w775 w786 w803 w812 w826 w835 w857 w871 w886 w896 w905 w929 w943 w961 w977 w986 w992 w1000 w1005 w1060 w1073] -> w652
          tunnel: w651 -> [_ _ _ _ _ _ _ _ _ w832 w841 w864 _ _ w902 _ _ _ w969 _ w985 w994 _ _ _ _]
          frame "TimeOut", Default {
          }
          frame "Close_Program" {
            w688 = T7 {"QueueAction"=enum."TimeOut", "Numeric 1"=0.0, "Numeric 2"=0.0, "Boolean 1"=FALSE, "Boolean 2"=FALSE, "Spin Program"=[], "Spin Prg v07"=[]}  # Device Queue
            n306 = Bundle By Name(cluster=w688, "QueueAction"=DeviceQueue_Action."Spectrometer_Close") -> (w683:T7)
            n307 = Bundle By Name(cluster=w683, "QueueAction"=DeviceQueue_Action."Laser_Close") -> (w681:T7)
            n308 = Bundle By Name(cluster=w681, "QueueAction"=DeviceQueue_Action."Arduino_Close") -> (w675:T7)
            n309 = Enqueue Element(queue=w687, element=w683, error in (no error)=w671) -> (queue out=w685:refnum<queue>, error out=w680:errorcluster)  [unwired: 1 in, 1 out]
            n310 = Bundle By Name(cluster=w675, "QueueAction"=DeviceQueue_Action."Close_Program") -> (w673:T7)
            n311 = Enqueue Element(queue=w685, element=w681, error in (no error)=w680) -> (queue out=w679:refnum<queue>, error out=w678:errorcluster)  [unwired: 1 in, 1 out]
            n312 = Enqueue Element(queue=w679, element=w675, error in (no error)=w678) -> (queue out=w677:refnum<queue>, error out=w676:errorcluster)  [unwired: 1 in, 1 out]
            n313 = Enqueue Element(queue=w677, element=w673, error in (no error)=w676) -> (queue out=w672:refnum<queue>, error out=w670:errorcluster)  [unwired: 1 in, 1 out]
            n314 = First Call?() -> (First Call?: T/F=w690:bool)
            n315 = Not(x=w690) -> (.not. x?=w689:bool)
          }
          frame "Abort" {
            w707 = T7 {"QueueAction"=enum."TimeOut", "Numeric 1"=0.0, "Numeric 2"=0.0, "Boolean 1"=FALSE, "Boolean 2"=FALSE, "Spin Program"=[], "Spin Prg v07"=[]}  # Device Queue
            n316 = Flush Queue(queue=w705, error in (no error)=w704) -> (queue out=w703:refnum<queue>, error out=w702:errorcluster)  [unwired: 1 out]
            n317 = Bundle By Name(cluster=w707, "QueueAction"=DeviceQueue_Action."Spectrometer_StopMeasurement") -> (w699:T7)
            n318 = Bundle By Name(cluster=w699, "QueueAction"=DeviceQueue_Action."Arduino_StopSpin") -> (w695:T7)
            n319 = Enqueue Element(queue=w703, element=w699, error in (no error)=w702) -> (queue out=w701:refnum<queue>, error out=w700:errorcluster)  [unwired: 1 in, 1 out]
            n320 = Bundle By Name(cluster=w695, "QueueAction"=DeviceQueue_Action."Measure_Stop") -> (w694:T7)
            n321 = Enqueue Element(queue=w701, element=w695, error in (no error)=w700) -> (queue out=w697:refnum<queue>, error out=w696:errorcluster)  [unwired: 1 in, 1 out]
            n322 = Enqueue Element(queue=w697, element=w694, error in (no error)=w696) -> (queue out=w691:refnum<queue>, error out=w692:errorcluster)  [unwired: 1 in, 1 out]
          }
          frame "Spectrometer_Init" {
            n323 = call-dynamic "Init.vi"("error in (no error)"=w725, "Variant"=0, "Avantes in"=refnum<class "Avantes.lvclass"> refnum ("Avantes.lvclass")) -> ("error out"=w724:errorcluster, "Avantes out"=w723:refnum<class "Avantes.lvclass">)  [unwired: 7 in]
            n324 = call-dynamic "IsInit.vi"("error in (no error)"=w724, "Avantes in"=w723) -> ("error out"=w720:errorcluster, "Is Init?"=w719:bool, "Avantes out"=w721:refnum<class "Avantes.lvclass">)  [unwired: 7 in]
            n325 = property on="Spectromter" class="Bool (strict)"("Value"=w719) -> ()  [unwired: 2 in, 2 out]
            n326 = property on="Init_Spectrometer" class="Bool (strict)"("Value"=w719) -> ()  [unwired: 2 in, 2 out]
            n327 = call-dynamic "Set_ExposurePerFrame.vi"("error in (no error)"=w720, "Exposure per Frame"=1, "Avantes in"=w721) -> ("error out"=w715:errorcluster, "Avantes out"=w718:refnum<class "Avantes.lvclass">)  [unwired: 7 in]
            n328 = case shown="True" w719 {
              tunnel: w718 -> [_ w741]
              tunnel: w715 -> [w730 w739]
              tunnel: [refnum<class "Abstract_CCD.lvclass"> refnum ("Abstract_CCD.lvclass") w740] -> w717
              tunnel: w714 -> [w731 w756]
              tunnel: [w731 w745] -> w713
              tunnel: [w730 w744] -> w712
              tunnel: w711 -> [w729 w736]
              tunnel: [w729 w734] -> w710
              frame False {
              }
              frame True {
                w742 = T5 {"QueueAction"=enum."TimeOut", "Data"=[], "Data_Raw"=[], "Data_Dark"=[], "Data_Ref"=[], "Device Information"=[], "Numeric Control"=0.0, "Boolean"=FALSE, "Wavelength"=[], "Time"=[], "Time Stamp"=timestamp(0 s since 1904-01-01), "Numeric Control 2"=0.0}  # DataQueue
                w757 = T7 {"QueueAction"=enum."TimeOut", "Numeric 1"=0.0, "Numeric 2"=0.0, "Boolean 1"=FALSE, "Boolean 2"=FALSE, "Spin Program"=[], "Spin Prg v07"=[]}  # Device Queue
                n329 = call-dynamic "Get_WavelengthAxis.vi"("error in (no error)"=w739, "Avantes in"=w741) -> ("error out"=w738:errorcluster, "lambda"=w733:dbl[unit][], "Avantes out"=w740:refnum<class "Avantes.lvclass">)  [unwired: 7 in]
                n330 = property on="Calculate Frames" class="Bool (strict)"() -> ("Value"=w749:bool)  [unwired: 2 in, 2 out]
                n331 = property on="Integration Time" class="DigNum (strict)"() -> ("Value"=w754:dbl[unit])  [unwired: 2 in, 2 out]
                n332 = Unbundle(w738) -> ("status"=w737:bool)  [unwired: 2 out]
                n333 = node(w754) -> (w753:dbl)
                n334 = Bundle By Name(cluster=w757, "QueueAction"=DeviceQueue_Action."Spectrometer_SetIntegrationTime", "Numeric 1"=w753, "Boolean 1"=w749) -> (w751:T7)
                n335 = property on="Frames" class="DigNum (strict)"() -> ("Value"=w748:i32)  [unwired: 2 in, 2 out]
                n336 = property on="Error_Spectromter" class="Bool (strict)"("Value"=w737) -> ()  [unwired: 2 in, 2 out]
                n337 = Enqueue Element(queue=w756, element=w751, error in (no error)=w739) -> (queue out=w752:refnum<queue>, error out=w746:errorcluster)  [unwired: 1 in, 1 out]
                n338 = Bundle By Name(cluster=w751, "QueueAction"=DeviceQueue_Action."Spectrometer_SetFrames", "Numeric 1"=w748) -> (w747:T7)
                n339 = Bundle By Name(cluster=w742, "QueueAction"=DataQueue_Action."Set_Wavelength", "Wavelength"=w733) -> (w743:T5)
                n340 = Enqueue Element(queue=w736, element=w743) -> (queue out=w734:refnum<queue>)  [unwired: 2 in, 2 out]
                n341 = Enqueue Element(queue=w752, element=w747, error in (no error)=w746) -> (queue out=w745:refnum<queue>, error out=w744:errorcluster)  [unwired: 1 in, 1 out]
              }
            }
            n342 = Bundle By Name(cluster=w722, "Abstract_CCD.lvclass"=w717) -> (w716:T4)
          }
          frame "Spectrometer_Close" {
            n343 = property on="Spectromter" class="Bool (strict)"("Value"=FALSE ("Spectromter")) -> ()  [unwired: 2 in, 2 out]
            n344 = Unbundle By Name(w763) -> ("Abstract_CCD.lvclass"=w766:refnum<class "Abstract_CCD.lvclass">)
            n345 = flat-sequence {
              tunnel: [refnum<class "Abstract_CCD.lvclass"> refnum ("Abstract_CCD.lvclass")] -> w760
              tunnel: w759 -> [_]
              frame #0 {
              }
            }
            n346 = call-dynamic "Close.vi"("error in (no error)"=w765, "Abstract_CCD in"=w766) -> ("error out"=w759:errorcluster)  [unwired: 8 in, 1 out]
            n347 = Bundle By Name(cluster=w763, "Abstract_CCD.lvclass"=w760) -> (w762:T4)
          }
          frame "Spectrometer_Measure" {
            w780 = T5 {"QueueAction"=enum."TimeOut", "Data"=[], "Data_Raw"=[], "Data_Dark"=[], "Data_Ref"=[], "Device Information"=[], "Numeric Control"=0.0, "Boolean"=FALSE, "Wavelength"=[], "Time"=[], "Time Stamp"=timestamp(0 s since 1904-01-01), "Numeric Control 2"=0.0}  # DataQueue
            n348 = Unbundle By Name(w775) -> ("Abstract_CCD.lvclass"=w779:refnum<class "Abstract_CCD.lvclass">)
            n349 = call-dynamic "Measure.vi"("error in (no error)"=w777, "Abstract_CCD in"=w779) -> ("error out"=w776:errorcluster, "Data Raw"=w770:T10, "Data"=w771:T10, "Darkspec"=w769:T10, "Time"=w768:dbl[])  [unwired: 3 in, 2 out]
            n350 = Bundle By Name(cluster=w780, "QueueAction"=DataQueue_Action."Spectrometer_Measure", "Data"=w771, "Data_Raw"=w770, "Data_Dark"=w769, "Time"=w768) -> (w781:T5)
            n351 = Enqueue Element(queue=w774, element=w781) -> (queue out=w773:refnum<queue>)  [unwired: 2 in, 2 out]
          }
          frame "Spectrometer_Preview" {
            w795 = T5 {"QueueAction"=enum."TimeOut", "Data"=[], "Data_Raw"=[], "Data_Dark"=[], "Data_Ref"=[], "Device Information"=[], "Numeric Control"=0.0, "Boolean"=FALSE, "Wavelength"=[], "Time"=[], "Time Stamp"=timestamp(0 s since 1904-01-01), "Numeric Control 2"=0.0}  # DataQueue
            n352 = Unbundle By Name(w787) -> ("Abstract_CCD.lvclass"=w785:refnum<class "Abstract_CCD.lvclass">)
            n353 = call-dynamic "Measure.vi"("error in (no error)"=w784, "Abstract_CCD in"=w785) -> ("error out"=w782:errorcluster, "Data Raw"=w792:T10, "Abstract_CCD out"=w783:refnum<class "Abstract_CCD.lvclass">)  [unwired: 3 in, 4 out]
            n354 = property on="Preview" class="Bool (strict)"(error in=w782) -> ("Value"=w790:bool)  [unwired: 1 in, 2 out]
            n355 = case shown="True" w790 {
              tunnel: [w797 w799] -> w789
              tunnel: w788 -> [w797 w798]
              frame False {
              }
              frame True {
                w801 = T7 {"QueueAction"=enum."TimeOut", "Numeric 1"=0.0, "Numeric 2"=0.0, "Boolean 1"=FALSE, "Boolean 2"=FALSE, "Spin Program"=[], "Spin Prg v07"=[]}  # Device Queue
                n356 = Bundle By Name(cluster=w801, "QueueAction"=DeviceQueue_Action."Spectrometer_Preview") -> (w800:T7)
                n357 = Enqueue Element(queue=w798, element=w800) -> (queue out=w799:refnum<queue>)  [unwired: 2 in, 2 out]
              }
            }
            n358 = Bundle By Name(cluster=w795, "Data_Raw"=w792, "QueueAction"=DataQueue_Action."Spectrometer_Preview") -> (w796:T5)
            n359 = Enqueue Element(queue=w794, element=w796) -> (queue out=w793:refnum<queue>)  [unwired: 2 in, 2 out]
            n360 = Bundle By Name(cluster=w787, "Abstract_CCD.lvclass"=w783) -> (w786:T4)
          }
          frame "Spectrometer_StartMeasurement" {
            n361 = Unbundle By Name(w805) -> ("Abstract_CCD.lvclass"=w809:refnum<class "Abstract_CCD.lvclass">)
            n362 = call-dynamic "StartMeasure.vi"("error in (no error)"=w810, "Frames"=-1, "Abstract_CCD in"=w809) -> ("error out"=w808:errorcluster, "Abstract_CCD out"=w804:refnum<class "Abstract_CCD.lvclass">)  [unwired: 7 in]
            n363 = Bundle By Name(cluster=w805, "Abstract_CCD.lvclass"=w804) -> (w803:T4)
          }
          frame "Spectrometer_StopMeasurement" {
            n364 = Unbundle By Name(w817) -> ("Abstract_CCD.lvclass"=w819:refnum<class "Abstract_CCD.lvclass">)
            n365 = call-dynamic "StopMeasurement.vi"("error in (no error)"=w818, "Abstract_CCD in"=w819) -> ("error out"=w815:errorcluster, "Abstract_CCD out"=w816:refnum<class "Abstract_CCD.lvclass">)  [unwired: 8 in]
            n366 = Bundle By Name(cluster=w817, "Abstract_CCD.lvclass"=w816) -> (w812:T4)
          }
          frame "Spectrometer_GetData" {
            w829 = T5 {"QueueAction"=enum."TimeOut", "Data"=[], "Data_Raw"=[], "Data_Dark"=[], "Data_Ref"=[], "Device Information"=[], "Numeric Control"=0.0, "Boolean"=FALSE, "Wavelength"=[], "Time"=[], "Time Stamp"=timestamp(0 s since 1904-01-01), "Numeric Control 2"=0.0}  # DataQueue
            n367 = Unbundle By Name(w826) -> ("Abstract_CCD.lvclass"=w831:refnum<class "Abstract_CCD.lvclass">)
            n368 = Unbundle By Name(w832) -> ("Numeric 1"=w823:dbl)
            n369 = call-dynamic "Measure_GetData.vi"("error in (no error)"=w830, "SpectraCount"=w823, "Abstract_CCD in"=w831) -> ("error out"=w820:errorcluster, "Data_Raw"=w822:T10, "Time"=w821:dbl[])  [unwired: 5 in, 1 out]
            n370 = Bundle By Name(cluster=w829, "QueueAction"=DataQueue_Action."Spectrometer_Measure", "Data_Raw"=w822, "Time"=w821) -> (w828:T5)
            n371 = Enqueue Element(queue=w825, element=w828) -> (queue out=w824:refnum<queue>)  [unwired: 2 in, 2 out]
          }
          frame "Spectrometer_SetIntegrationTime" {
            n372 = Unbundle By Name(w841) -> ("Numeric 1"=w843:dbl)
            n373 = Unbundle By Name(w837) -> ("Abstract_CCD.lvclass"=w845:refnum<class "Abstract_CCD.lvclass">)
            n374 = Unbundle By Name(w841) -> ("Boolean 1"=w840:bool)
            n375 = node(w843) -> (w842:dbl[unit])
            n376 = call-dynamic "Set_ExposureTime.vi"("error in (no error)"=w844, "Exposure Time"=w842, "Abstract_CCD in"=w845) -> ("error out"=w848:errorcluster, "Abstract_CCD out"=w847:refnum<class "Abstract_CCD.lvclass">)  [unwired: 7 in]
            n377 = call-dynamic "Get_FrameRate.vi"("error in (no error)"=w848, "Abstract_CCD in"=w847) -> ("error out"=w838:errorcluster, "Frame Rate"=w839:dbl[unit], "Abstract_CCD out"=w836:refnum<class "Abstract_CCD.lvclass">)  [unwired: 7 in]
            "Frame Rate" <- w839
            n378 = Bundle By Name(cluster=w837, "Abstract_CCD.lvclass"=w836) -> (w835:T4)
            n379 = case shown="True" w840 {
              tunnel: w839 -> [_ w852]
              frame False {
              }
              frame True {
                n380 = property on="Program Spin Coater" class="Arr (strict)"() -> ("Value"=w849:T1)  [unwired: 2 in, 2 out]
                n381 = property on="Seconds to Spin Start" class="DigNum (strict)"() -> ("Value"=w854:dbl[unit])  [unwired: 2 in, 2 out]
                n382 = property on="Seconds after Spin Stop" class="DigNum (strict)"() -> ("Value"=w853:dbl[unit])  [unwired: 2 in, 2 out]
                n383 = call "CalculateFrames_v02.vi"("Program Spin Coater"=w849, "Seconds End"=w853, "Seconds Start"=w854, "Frame Rate"=w852) -> ("Time"=w851:dbl, "Frames"=w850:i32)  [unwired: 6 in]
                n384 = property on="Overall Time" class="DigNum (strict)"("Value"=w851) -> ()  [unwired: 2 in, 2 out]
                n385 = property on="Frames" class="DigNum (strict)"("Value"=w850) -> ()  [unwired: 2 in, 2 out]
              }
            }
          }
          frame "Spectrometer_SetFrames" {
            n386 = Unbundle By Name(w856) -> ("Abstract_CCD.lvclass"=w861:refnum<class "Abstract_CCD.lvclass">)
            n387 = Unbundle By Name(w864) -> ("Numeric 1"=w858:dbl)
            n388 = call-dynamic "Set_Frames.vi"("error in (no error)"=w860, "Frames"=w858, "Abstract_CCD in"=w861) -> ("error out"=w859:errorcluster, "Abstract_CCD out"=w855:refnum<class "Abstract_CCD.lvclass">)  [unwired: 7 in]
            n389 = Bundle By Name(cluster=w856, "Abstract_CCD.lvclass"=w855) -> (w857:T4)
          }
          frame "Spectrometer_SetDarkspec" {
            w877 = T5 {"QueueAction"=enum."TimeOut", "Data"=[], "Data_Raw"=[], "Data_Dark"=[], "Data_Ref"=[], "Device Information"=[], "Numeric Control"=0.0, "Boolean"=FALSE, "Wavelength"=[], "Time"=[], "Time Stamp"=timestamp(0 s since 1904-01-01), "Numeric Control 2"=0.0}  # DataQueue
            n390 = Unbundle By Name(w872) -> ("Abstract_CCD.lvclass"=w870:refnum<class "Abstract_CCD.lvclass">)
            n391 = call-dynamic "Measure.vi"("error in (no error)"=w869, "Abstract_CCD in"=w870) -> ("error out"=w867:errorcluster, "Data Raw"=w874:T10, "Abstract_CCD out"=w868:refnum<class "Abstract_CCD.lvclass">)  [unwired: 3 in, 4 out]
            n392 = Bundle By Name(cluster=w877, "QueueAction"=DataQueue_Action."Set_Dark", "Data_Dark"=w874) -> (w878:T5)
            n393 = Enqueue Element(queue=w876, element=w878) -> (queue out=w873:refnum<queue>)  [unwired: 2 in, 2 out]
            n394 = Bundle By Name(cluster=w872, "Abstract_CCD.lvclass"=w868) -> (w871:T4)
            n395 = property on="Record_Darkspec" class="Bool (strict)"(error in=w867, "Value"=FALSE ("Record_Darkspec")) -> (error out=w866:errorcluster)  [unwired: 1 in, 1 out]
          }
          frame "Spectrometer_SetReference" {
            w892 = T5 {"QueueAction"=enum."TimeOut", "Data"=[], "Data_Raw"=[], "Data_Dark"=[], "Data_Ref"=[], "Device Information"=[], "Numeric Control"=0.0, "Boolean"=FALSE, "Wavelength"=[], "Time"=[], "Time Stamp"=timestamp(0 s since 1904-01-01), "Numeric Control 2"=0.0}  # DataQueue
            n396 = Unbundle By Name(w887) -> ("Abstract_CCD.lvclass"=w884:refnum<class "Abstract_CCD.lvclass">)
            n397 = call-dynamic "Measure.vi"("error in (no error)"=w885, "Abstract_CCD in"=w884) -> ("error out"=w882:errorcluster, "Data Raw"=w889:T10, "Abstract_CCD out"=w883:refnum<class "Abstract_CCD.lvclass">)  [unwired: 3 in, 4 out]
            n398 = Bundle By Name(cluster=w892, "QueueAction"=DataQueue_Action."Set_Ref", "Data_Ref"=w889) -> (w893:T5)
            n399 = Enqueue Element(queue=w891, element=w893) -> (queue out=w888:refnum<queue>)  [unwired: 2 in, 2 out]
            n400 = Bundle By Name(cluster=w887, "Abstract_CCD.lvclass"=w883) -> (w886:T4)
            n401 = property on="Record RefSpec" class="Bool (strict)"(error in=w882, "Value"=FALSE ("Record RefSpec")) -> (error out=w881:errorcluster)  [unwired: 1 in, 1 out]
          }
          frame "Spectrometer_SetTriggerMode" {
            n402 = Unbundle By Name(w898) -> ("Abstract_CCD.lvclass"=w903:refnum<class "Abstract_CCD.lvclass">)
            n403 = Unbundle By Name(w902) -> ("Numeric 1"=w900:dbl)
            n404 = call-dynamic "Set_TriggerMode.vi"("error in (no error)"=w901, "Trigger Mode"=w900, "Abstract_CCD in"=w903) -> ("error out"=w899:errorcluster, "Abstract_CCD out"=w897:refnum<class "Abstract_CCD.lvclass">)  [unwired: 7 in]
            n405 = Bundle By Name(cluster=w898, "Abstract_CCD.lvclass"=w897) -> (w896:T4)
          }
          frame "Spectrometer_DeviceInformation" {
            w911 = T5 {"QueueAction"=enum."TimeOut", "Data"=[], "Data_Raw"=[], "Data_Dark"=[], "Data_Ref"=[], "Device Information"=[], "Numeric Control"=0.0, "Boolean"=FALSE, "Wavelength"=[], "Time"=[], "Time Stamp"=timestamp(0 s since 1904-01-01), "Numeric Control 2"=0.0}  # DataQueue
            n406 = Unbundle By Name(w905) -> ("Abstract_CCD.lvclass"=w913:refnum<class "Abstract_CCD.lvclass">)
            n407 = call-dynamic "Get_DeviceInformation.vi"("error in (no error)"=w912, "Abstract_CCD in"=w913) -> ("error out"=w907:errorcluster, "Array"=w914:string[])  [unwired: 7 in, 1 out]
            n408 = Bundle By Name(cluster=w911, "QueueAction"=DataQueue_Action."Transfer_Settings", "Device Information"=w914) -> (w909:T5)
            n409 = Enqueue Element(queue=w910, element=w909, error in (no error)=w907) -> (queue out=w908:refnum<queue>, error out=w906:errorcluster)  [unwired: 1 in, 1 out]
          }
          frame "Arduino_Init" {
            n410 = Unbundle By Name(w925) -> ("SpinCoater.lvclass"=w924:refnum<class "SpinCoater.lvclass">)
            n411 = call-dynamic "Init.vi"("error in (no error)"=w923, "Variant"="Port Arduino", "SpinCoater in"=w924) -> ("error out"=w920:errorcluster, "SpinCoater out"=w921:refnum<class "SpinCoater.lvclass">)  [unwired: 7 in]
            n412 = call-dynamic "IsInit.vi"("error in (no error)"=w920, "SpinCoater in"=w921) -> ("error out"=w917:errorcluster, "Init"=w918:bool, "SpinCoater out"=w919:refnum<class "SpinCoater.lvclass">)  [unwired: 7 in]
            n413 = property on="Arduino" class="Bool (strict)"("Value"=w918) -> ()  [unwired: 2 in, 2 out]
            n414 = case shown="True" w918 {
              tunnel: w928 -> [w932 w941]
              tunnel: [w932 w935] -> w927
              tunnel: [w931 w934] -> w926
              tunnel: w917 -> [w931 w938]
              frame False {
              }
              frame True {
                w942 = T7 {"QueueAction"=enum."TimeOut", "Numeric 1"=0.0, "Numeric 2"=0.0, "Boolean 1"=FALSE, "Boolean 2"=FALSE, "Spin Program"=[], "Spin Prg v07"=[]}  # Device Queue
                n415 = property on="Program Spin Coater" class="Arr (strict)"() -> ("Value"=w933:T1)  [unwired: 2 in, 2 out]
                n416 = property on="Seconds to Spin Start" class="DigNum (strict)"() -> ("Value"=w937:dbl[unit])  [unwired: 2 in, 2 out]
                n417 = node(w937) -> (w936:dbl)
                n418 = Bundle By Name(cluster=w942, "QueueAction"=DeviceQueue_Action."Arduino_LoadProgram", "Spin Prg v07"=w933, "Numeric 1"=w936) -> (w940:T7)
                n419 = Enqueue Element(queue=w941, element=w940, error in (no error)=w938) -> (queue out=w935:refnum<queue>, error out=w934:errorcluster)  [unwired: 1 in, 1 out]
              }
            }
            n420 = Bundle By Name(cluster=w925, "SpinCoater.lvclass"=w919) -> (w929:T4)
          }
          frame "Arduino_Close" {
            n421 = Unbundle By Name(w945) -> ("SpinCoater.lvclass"=w953:refnum<class "SpinCoater.lvclass">)
            n422 = property on="Arduino" class="Bool (strict)"() -> (error out=w947:errorcluster, "Value"=w946:bool)  [unwired: 2 in, 1 out]
            n423 = property on="Arduino" class="Bool (strict)"(error in=w947, "Value"=FALSE ("Arduino")) -> ()  [unwired: 1 in, 2 out]
            n424 = case shown="False" w946 {
              tunnel: w953 -> [w954 w959]
              tunnel: w952 -> [w955 w958]
              tunnel: [w955 w957] -> w951
              tunnel: [w954 w956] -> w944
              frame False {
              }
              frame True {
                n425 = call-dynamic "Close.vi"("error in (no error)"=w958, "SpinCoater in"=w959) -> ("error out"=w957:errorcluster, "SpinCoater out"=w956:refnum<class "SpinCoater.lvclass">)  [unwired: 8 in]
              }
            }
            n426 = Bundle By Name(cluster=w945, "SpinCoater.lvclass"=w944) -> (w943:T4)
          }
          frame "Arduino_LoadProgram" {
            n427 = Unbundle By Name(w969) -> ("Spin Prg v07"=w960:T1, "Numeric 1"=w968:dbl)
            n428 = Unbundle By Name(w964) -> ("SpinCoater.lvclass"=w967:refnum<class "SpinCoater.lvclass">)
            n429 = node(w968) -> (w966:dbl[unit])
            n430 = call-dynamic "Program_Load_v02.vi"("error in (no error)"=w965, "Time Start"=w966, "Program Spin Coater"=w960, "SpinCoater in"=w967) -> ("error out"=w962:errorcluster, "SpinCoater out"=w963:refnum<class "SpinCoater.lvclass">)  [unwired: 6 in]
            n431 = Bundle By Name(cluster=w964, "SpinCoater.lvclass"=w963) -> (w961:T4)
          }
          frame "Arduino_StartProgram" {
            n432 = Unbundle By Name(w977) -> ("SpinCoater.lvclass"=w974:refnum<class "SpinCoater.lvclass">)
            n433 = call-dynamic "Program_Run.vi"("error in (no error)"=w973, "SpinCoater in"=w974) -> ("error out"=w972:errorcluster)  [unwired: 8 in, 1 out]
            n434 = property on="Action" class="Str"("Value"="Measuring" ("Action")) -> ()  [unwired: 2 in, 2 out]
          }
          frame "Arduino_SetSpeed" {
            n435 = Unbundle By Name(w986) -> ("SpinCoater.lvclass"=w982:refnum<class "SpinCoater.lvclass">)
            n436 = Unbundle By Name(w985) -> ("Numeric 1"=w984:dbl)
            n437 = To Unsigned Long Integer(number=w984) -> (unsigned 32bit integer=w980:u32)
            n438 = call-dynamic "Debug_SetSpeed.vi"("error in (no error)"=w981, "Speed"=w980, "SpinCoater in"=w982) -> ("error out"=w979:errorcluster)  [unwired: 7 in, 1 out]
          }
          frame "Arduino_SetMillis" {
            n439 = Unbundle By Name(w992) -> ("SpinCoater.lvclass"=w991:refnum<class "SpinCoater.lvclass">)
            n440 = Unbundle By Name(w994) -> ("Numeric 1"=w996:dbl)
            n441 = To Unsigned Long Integer(number=w996) -> (unsigned 32bit integer=w988:u32)
            n442 = call-dynamic "Debug_SetMillis.vi"("error in (no error)"=w990, "Milliseconds"=w988, "SpinCoater in"=w991) -> ("error out"=w989:errorcluster)  [unwired: 7 in, 1 out]
          }
          frame "Arduino_StopSpin" {
            n443 = Unbundle By Name(w1000) -> ("SpinCoater.lvclass"=w999:refnum<class "SpinCoater.lvclass">)
            n444 = call-dynamic "Stop_Spin.vi"("error in (no error)"=w998, "SpinCoater in"=w999) -> ("error out"=w997:errorcluster)  [unwired: 8 in, 1 out]
          }
          frame "Measure_Stop" {
            w1009 = T5 {"QueueAction"=enum."TimeOut", "Data"=[], "Data_Raw"=[], "Data_Dark"=[], "Data_Ref"=[], "Device Information"=[], "Numeric Control"=0.0, "Boolean"=FALSE, "Wavelength"=[], "Time"=[], "Time Stamp"=timestamp(0 s since 1904-01-01), "Numeric Control 2"=0.0}  # DataQueue
            n445 = Bundle By Name(cluster=w1009, "QueueAction"=DataQueue_Action."Stop_Measurement") -> (w1010:T5)
            n446 = Enqueue Element(queue=w1007, element=w1010, error in (no error)=w1004) -> (queue out=w1006:refnum<queue>, error out=w1003:errorcluster)  [unwired: 1 in, 1 out]
          }
          frame "Measure_InSitu" {
            w1051 = T7 {"QueueAction"=enum."TimeOut", "Numeric 1"=0.0, "Numeric 2"=0.0, "Boolean 1"=FALSE, "Boolean 2"=FALSE, "Spin Program"=[], "Spin Prg v07"=[]}  # Device Queue
            w1058 = T7 {"QueueAction"=enum."TimeOut", "Numeric 1"=0.0, "Numeric 2"=0.0, "Boolean 1"=FALSE, "Boolean 2"=FALSE, "Spin Program"=[], "Spin Prg v07"=[]}  # Device Queue
            n447 = Bundle By Name(cluster=w1058, "QueueAction"=DeviceQueue_Action."Spectrometer_SetTriggerMode", "Numeric 1"=1.0) -> (w1056:T7)
            n448 = Bundle By Name(cluster=w1051, "QueueAction"=DeviceQueue_Action."Spectrometer_DeviceInformation") -> (w1048:T7)
            n449 = Bundle By Name(cluster=w1048, "QueueAction"=DeviceQueue_Action."Spectrometer_StartMeasurement") -> (w1044:T7)
            n450 = Enqueue Element(queue=w1057, element=w1056, error in (no error)=w1013) -> (queue out=w1053:refnum<queue>, error out=w1054:errorcluster)  [unwired: 1 in, 1 out]
            n451 = property on="Frames" class="DigNum (strict)"() -> ("Value"=w1014:i32)  [unwired: 2 in, 2 out]
            n452 = Bundle By Name(cluster=w1044, "QueueAction"=DeviceQueue_Action."Arduino_StartProgram") -> (w1039:T7)
            n453 = Enqueue Element(queue=w1053, element=w1048, error in (no error)=w1054) -> (queue out=w1050:refnum<queue>, error out=w1049:errorcluster)  [unwired: 1 in, 1 out]
            n454 = Bundle By Name(cluster=w1039, "QueueAction"=DeviceQueue_Action."Spectrometer_GetData", "Numeric 1"="Dividider Get Spectra") -> (w1034:T7)
            n455 = Divide(x=w1014, y="Dividider Get Spectra") -> (x/y=w1046:dbl)
            n456 = Round Toward +Infinity(x=w1046) -> (ceil(x): smallest int >= x=w1045:dbl)
            n457 = Enqueue Element(queue=w1050, element=w1044, error in (no error)=w1049) -> (queue out=w1043:refnum<queue>, error out=w1042:errorcluster)  [unwired: 1 in, 1 out]
            n458 = Enqueue Element(queue=w1043, element=w1039, error in (no error)=w1042) -> (queue out=w1040:refnum<queue>, error out=w1037:errorcluster)  [unwired: 1 in, 1 out]
            n459 = for {
              N: w1045 -> [_]
              shift-right: [w1061] -> w1036
              shift-left: w1040 -> [w1065]
              tunnel: w1034 -> [w1062]
              shift-right: [w1063] -> w1035
              shift-left: w1037 -> [w1064]
              n460 = Enqueue Element(queue=w1065, element=w1062, error in (no error)=w1064) -> (queue out=w1061:refnum<queue>, error out=w1063:errorcluster)  [unwired: 1 in, 1 out]
            }
            n461 = Bundle By Name(cluster=w1034, "QueueAction"=DeviceQueue_Action."Spectrometer_StopMeasurement") -> (w1030:T7)
            n462 = property on="Frames for Spectrometer" class="DigNum (strict)"() -> ("Value"=w1016:dbl)  [unwired: 2 in, 2 out]
            n463 = Bundle By Name(cluster=w1030, "QueueAction"=DeviceQueue_Action."Measure_Stop") -> (w1023:T7)
            n464 = Enqueue Element(queue=w1036, element=w1030, error in (no error)=w1035) -> (queue out=w1031:refnum<queue>, error out=w1032:errorcluster)  [unwired: 1 in, 1 out]
            n465 = Bundle By Name(cluster=w1023, "QueueAction"=DeviceQueue_Action."Spectrometer_SetTriggerMode", "Numeric 1"=0.0) -> (w1018:T7)
            n466 = Enqueue Element(queue=w1031, element=w1023, error in (no error)=w1032) -> (queue out=w1026:refnum<queue>, error out=w1027:errorcluster)  [unwired: 1 in, 1 out]
            n467 = Bundle By Name(cluster=w1018, "QueueAction"=DeviceQueue_Action."Spectrometer_SetFrames", "Numeric 1"=w1016) -> (w1015:T7)
            n468 = Enqueue Element(queue=w1026, element=w1018, error in (no error)=w1027) -> (queue out=w1025:refnum<queue>, error out=w1024:errorcluster)  [unwired: 1 in, 1 out]
            n469 = Enqueue Element(queue=w1025, element=w1015, error in (no error)=w1024) -> (queue out=w1019:refnum<queue>, error out=w1020:errorcluster)  [unwired: 1 in, 1 out]
          }
          frame "Measure_Spectrum" {
            w1078 = T7 {"QueueAction"=enum."TimeOut", "Numeric 1"=0.0, "Numeric 2"=0.0, "Boolean 1"=FALSE, "Boolean 2"=FALSE, "Spin Program"=[], "Spin Prg v07"=[]}  # Device Queue
            n470 = Bundle By Name(cluster=w1078, "QueueAction"=DeviceQueue_Action."Spectrometer_Measure") -> (w1070:T7)
            n471 = Bundle By Name(cluster=w1070, "QueueAction"=DeviceQueue_Action."Measure_Stop") -> (w1068:T7)
            n472 = Enqueue Element(queue=w1076, element=w1070, error in (no error)=w1075) -> (queue out=w1071:refnum<queue>, error out=w1072:errorcluster)  [unwired: 1 in, 1 out]
            n473 = Enqueue Element(queue=w1071, element=w1068, error in (no error)=w1072) -> (queue out=w1067:refnum<queue>, error out=w1066:errorcluster)  [unwired: 1 in, 1 out]
          }
        }
      }
      frame Error {
        w1083 = T15 4 items=["no dialog", "OK message", "continue or stop message", "OK message + warnings", "continue/stop + warnings"] ("type of dialog (OK msg:1)")
        n474 = call <vilib>:"General Error Handler.vi"("type of dialog (OK msg:1)"=w1083, "error in (no error)"=w1084) -> ("error out"=w1082:errorcluster)  [unwired: 9 in, 4 out]
        n475 = call <vilib>:"Clear Errors.vi"("error in (no error)"=w1082) -> ("error out"=w1081:errorcluster)  [unwired: 5 in, 1 out]
      }
    }
  }
  n476 = disable-structure shown="Disabled" {
    frame Disabled {
      w1087 = T7 {"QueueAction"=enum."TimeOut", "Numeric 1"=0.0, "Numeric 2"=0.0, "Boolean 1"=FALSE, "Boolean 2"=FALSE, "Spin Program"=[], "Spin Prg v07"=[]}  # Device Queue
      n477 = Bundle By Name(cluster=w1087, "QueueAction"=DeviceQueue_Action."Arduino_SetSpeed") -> (w1086:T7)  [unwired: 1 in]
      n478 = Enqueue Element(element=w1086) -> ()  [unwired: 3 in, 3 out]
    }
    frame Enabled {
    }
  }
  n479 = Release Queue(queue=w9) -> ()  [unwired: 2 in, 3 out]
  n480 = Release Queue(queue=w10) -> ()  [unwired: 2 in, 3 out]
